vi "EELS Test V3.vi"() -> ()   [LabVIEW 2012]
uses:
  <instrlib>/Quantum Composers 9000 Series/Quantum Composers 9000 Series.lvlib
panel:
  in  "Continuous Wave":bool=TRUE
  out "Spectrum Measurement Recipe ID":dbl
  out "Dates":T1={"Measurement Date"=timestamp(3619697085.7529235 s since 1904-01-01), "Session Date"=timestamp(0 s since 1904-01-01)}
  in  "DeviceInfo":T2={"Cavity Length (um)"="1500", "Cavity Width (um)"="10", "X Position"="1", "Part Name"="0-0-1-10-1500"}
  out "Processing Recipe ID":dbl
  out "Spectrum Parameters":T3={"Peak Wavelengh (dbm)"="", "Peak Power (dbm)"="", "FWHM (nm)"="", "Input Current (mA)"="", "Measurement Recipe ID"=1.0, "Processing Recipe ID"=0.0, "Temperature"=0.0}
  out "LIV Array":dbl[][](array[numeric])=[[1.304, 1.304, 1.304, 1.304, 1.304, 1.304, 1.304, 1.303, 1.303, 1.302, 1.302, 1.302, 1.302, 1.302, 1.301, 1.301, 1.301, 1.301, 1.3, 1.3, 1.3, 1.3, 1.299, 1.299, 1.3, 1.299, 1.299, 1.298, 1.298, 1.298, 1.298, 1.296, 1.296, 1.296, 1.296, 1.296, 1.295, 1.295, 1.295, 1.295, 1.294, 1.294, 1.294, 1.294, 1.294, 1.292, 1.292, 1.292, 1.292, 1.29, 1.29, 1.29, 1.29, 1.29, 1.289, 1.289, 1.289, 1.289, 1.288, 1.287, 1.287, 1.287, 1.285, 1.285, 1.285, 1.285, 1.285, 1.283, 1.283, 1.283, 1.284, 1.282, 1.282, 1.282, 1.282, 1.282, 1.28, 1.28, 1.28, 1.28, 1.28, 1.278, 1.278, 1.278, 1.278, 1.276, 1.276, 1.276, 1.276, 1.274, 1.274, 1.274, 1.274, 1.274, 1.272, 1.272, 1.272, 1.272, 1.269, 1.269, 1.269, 1.269, 1.269, 1.267, 1.267, 1.267, 1.268, 1.265, 1.265, 1.265, 1.265, 1.265, 1.263, 1.263, 1.263, 1.263, 1.261, 1.261, 1.261, 1.261, 1.261, 1.259, 1.259, 1.259, 1.259, 1.256, 1.256, 1.256, 1.256, 1.256, 1.254, 1.254, 1.254, 1.254, 1.252, 1.252, 1.252, 1.252, 1.25, 1.249, 1.249, 1.249, 1.249, 1.248, 1.248, 1.248, 1.247, 1.245, 1.245, 1.245, 1.245, 1.245, 1.243, 1.243, 1.243, 1.243, 1.241, 1.241, 1.241, 1.241, 1.241, 1.238, 1.238, 1.238, 1.238, 1.236, 1.236, 1.236, 1.236, 1.236, 1.234, 1.234, 1.234, 1.234, 1.232, 1.232, 1.232, 1.232, 1.229, 1.229, 1.229, 1.229, 1.229, 1.227, 1.227, 1.227, 1.227, 1.227, 1.225, 1.225, 1.225, 1.225, 1.223, 1.223, 1.222, 1.223, 1.223, 1.22, 1.22, 1.22, 1.22], [216.66666666666669, 216.66666666666669, 216.66666666666669, 216.66666666666669, 216.66666666666669, 220.0, 220.0, 220.0, 220.0, 223.33333333333334, 226.66666666666666, 226.66666666666666, 223.33333333333334, 223.33333333333334, 230.00000000000003, 230.00000000000003, 230.00000000000003, 230.00000000000003, 233.33333333333334, 233.33333333333334, 233.33333333333334, 233.33333333333334, 236.66666666666666, 236.66666666666666, 236.66666666666666, 236.66666666666666, 236.66666666666666, 243.33333333333334, 243.33333333333334, 243.33333333333334, 243.33333333333334, 246.66666666666669, 246.66666666666669, 246.66666666666669, 246.66666666666669, 246.66666666666669, 250.0, 250.0, 250.0, 250.0, 256.6666666666667, 256.6666666666667, 256.6666666666667, 256.6666666666667, 256.6666666666667, 260.0, 260.0, 260.0, 260.0, 263.33333333333337, 263.33333333333337, 263.33333333333337, 263.33333333333337, 263.33333333333337, 270.0, 270.0, 270.0, 270.0, 273.3333333333333, 273.3333333333333, 273.3333333333333, 273.3333333333333, 276.6666666666667, 276.6666666666667, 276.6666666666667, 276.6666666666667, 276.6666666666667, 283.33333333333337, 283.33333333333337, 280.0, 283.33333333333337, 286.6666666666667, 286.6666666666667, 286.6666666666667, 286.6666666666667, 286.6666666666667, 290.0, 290.0, 290.0, 290.0, 290.0, 293.33333333333337, 293.33333333333337, 293.33333333333337, 293.33333333333337, 300.0, 300.0, 300.0, 300.0, 303.3333333333333, 303.3333333333333, 303.3333333333333, 303.3333333333333, 303.3333333333333, 306.66666666666663, 306.66666666666663, 306.66666666666663, 306.66666666666663, 313.33333333333337, 313.33333333333337, 313.33333333333337, 313.33333333333337, 313.33333333333337, 316.6666666666667, 316.6666666666667, 316.6666666666667, 316.6666666666667, 320.0, 320.0, 320.0, 320.0, 320.0, 326.6666666666667, 326.6666666666667, 326.6666666666667, 326.6666666666667, 330.0, 330.0, 330.0, 330.0, 330.0, 333.33333333333337, 333.33333333333337, 333.33333333333337, 333.33333333333337, 340.0, 340.0, 340.0, 340.0, 340.0, 343.33333333333337, 343.33333333333337, 343.33333333333337, 343.33333333333337, 346.6666666666667, 346.6666666666667, 346.6666666666667, 346.6666666666667, 353.3333333333333, 353.3333333333333, 353.3333333333333, 353.3333333333333, 353.3333333333333, 356.66666666666663, 356.66666666666663, 356.66666666666663, 356.66666666666663, 360.00000000000006, 360.00000000000006, 360.00000000000006, 360.00000000000006, 360.00000000000006, 363.33333333333337, 363.33333333333337, 363.33333333333337, 363.33333333333337, 370.0, 370.0, 370.0, 370.0, 370.0, 373.3333333333333, 373.3333333333333, 373.3333333333333, 373.3333333333333, 376.6666666666667, 376.6666666666667, 376.6666666666667, 376.6666666666667, 376.6666666666667, 383.33333333333337, 383.33333333333337, 383.33333333333337, 383.33333333333337, 386.6666666666667, 386.6666666666667, 386.6666666666667, 386.6666666666667, 390.0, 390.0, 390.0, 390.0, 390.0, 396.6666666666667, 396.6666666666667, 396.6666666666667, 396.6666666666667, 396.6666666666667, 400.0, 400.0, 400.0, 400.0, 406.6666666666667, 403.3333333333333, 403.3333333333333, 403.3333333333333, 403.3333333333333, 410.00000000000006, 410.00000000000006, 410.00000000000006, 410.00000000000006], [0.025723833333333338, 0.025771333333333334, 0.025723833333333338, 0.025700133333333337, 0.025723833333333338, 0.02764603333333333, 0.02766973333333333, 0.02764603333333333, 0.02766973333333333, 0.029568200000000003, 0.029568200000000003, 0.0295207, 0.029568200000000003, 0.0295919, 0.0316802, 0.0316802, 0.0316802, 0.03165646666666667, 0.03395833333333333, 0.03393466666666667, 0.03393466666666667, 0.033982000000000005, 0.036331333333333334, 0.036331333333333334, 0.036355000000000005, 0.036355000000000005, 0.03630766666666667, 0.038941666666666666, 0.039013, 0.038941666666666666, 0.03896533333333333, 0.041931666666666666, 0.041931666666666666, 0.041931666666666666, 0.041979333333333334, 0.042003, 0.04549133333333334, 0.04549133333333334, 0.04542, 0.04546766666666667, 0.050190000000000005, 0.050166333333333334, 0.050166333333333334, 0.050095, 0.05011866666666667, 0.05785466666666667, 0.057926, 0.05783100000000001, 0.05785466666666667, 0.094637, 0.09451833333333334, 0.09373533333333334, 0.09423366666666667, 0.094281, 0.259421, 0.26146166666666665, 0.26518733333333333, 0.2657333333333333, 0.5063133333333334, 0.5069066666666667, 0.51006, 0.50268, 0.7989800000000001, 0.7944466666666667, 0.7896766666666666, 0.7862133333333332, 0.78664, 1.13296, 1.1350733333333334, 1.1380633333333332, 1.1477933333333334, 1.4813300000000003, 1.48841, 1.4895933333333333, 1.4940766666666667, 1.48912, 1.9095566666666668, 1.90578, 1.8970466666666668, 1.89445, 1.8982266666666667, 2.34109, 2.3356600000000003, 2.3382566666666666, 2.3389666666666664, 2.81795, 2.83778, 2.8368333333333333, 2.8559566666666667, 3.3503000000000003, 3.344866666666667, 3.341066666666667, 3.3392, 3.335633333333333, 3.8592333333333335, 3.864666666666667, 3.8618333333333337, 3.8595, 4.399366666666667, 4.393933333333333, 4.3963, 4.397966666666667, 4.399133333333333, 4.958866666666666, 4.962166666666667, 4.9761, 4.977733333333334, 5.538166666666667, 5.536033333333334, 5.5365, 5.5436, 5.5311, 6.106366666666666, 6.103800000000001, 6.095766666666667, 6.0974, 6.676966666666666, 6.6828666666666665, 6.690433333333333, 6.687600000000001, 6.693966666666666, 7.294766666666667, 7.293333333333333, 7.291666666666667, 7.287433333333334, 7.871233333333334, 7.878066666666667, 7.8729000000000005, 7.8729000000000005, 7.864633333333334, 8.461866666666667, 8.467766666666668, 8.455266666666667, 8.465900000000001, 9.044733333333333, 9.0492, 9.0622, 9.052033333333336, 9.645299999999999, 9.661566666666666, 9.650966666666669, 9.659433333333334, 9.656866666666666, 10.165566666666667, 10.169366666666667, 10.176666666666668, 10.1781, 10.767566666666667, 10.786433333333335, 10.7666, 10.7678, 10.763766666666665, 11.351833333333333, 11.3431, 11.329166666666666, 11.334833333333334, 11.923100000000002, 11.913666666666668, 11.905166666666666, 11.904933333333334, 11.9002, 12.472433333333333, 12.484966666666669, 12.479066666666666, 12.474100000000002, 13.1072, 13.093033333333334, 13.1072, 13.121366666666669, 13.097766666666667, 13.723166666666668, 13.711366666666667, 13.6854, 13.718433333333333, 14.334400000000002, 14.315500000000002, 14.282466666666666, 14.308433333333333, 14.988100000000001, 14.929100000000002, 14.947966666666668, 14.962133333333334, 14.933800000000002, 15.799900000000001, 15.788133333333334, 15.804633333333333, 15.804633333333333, 15.764533333333334, 16.9209, 16.939766666666667, 16.9445, 16.913833333333333, 17.938033333333333, 17.869600000000002, 17.909733333333335, 17.8932, 17.900266666666663, 18.6838, 18.6413, 18.672, 18.620066666666666]]
  in  "Operator":string="sswifter"
  out "LIV Parameters":T4={"Threshold Current (mA)"=0.0, "Threshold Voltage (V)"=1.288, "Slope Efficiency"=1.0882708585247884, "Temperature"=15.0, "Measurement Recipe ID"=1.0, "Processing Recipe ID"=0.0}
  in  "update wafer info":bool
  in  "WaferInfo":T5={"WaferName"="TGR-163-1", "Scribe"="J3393-115", "Structure"="1068.1.1", "Lot"="SJC_ENG_375_4-GaAs", "Mask"="PH002"}
  in  "vi find peak":path=path "C:/Users/test_QE/Desktop/NanoMAX SubVI/NanoMAX 1D Find Peak Power 3D.vi"
  in  "vi path piezosfine":path=path "C:/Users/test_QE/Desktop/NanoMAX SubVI/NanoMAX300 Align Fiber Piezos.vi"
  in  "vi path stepper fine":path=path "C:/Users/test_QE/Desktop/NanoMAX SubVI/NanoMAX300 Align Fiber Steppers.vi"
  out "intensity array":dbl[](array[numeric])
  out "Wavelength Array":dbl[](array[numeric])
  out "data step":dbl
  out "Current lambda":dbl
  out "Numeric":i32
  out "Piezo Refs":refnum<k7>[](array[refnum])
  out "Stepper Refs":refnum<k7>[](array[refnum])
  in  "stop":bool
  out "P array":dbl[](array[numeric])=[0.025723833333333338, 0.025771333333333334, 0.025723833333333338, 0.025700133333333337, 0.025723833333333338, 0.02764603333333333, 0.02766973333333333, 0.02764603333333333, 0.02766973333333333, 0.029568200000000003, 0.029568200000000003, 0.0295207, 0.029568200000000003, 0.0295919, 0.0316802, 0.0316802, 0.0316802, 0.03165646666666667, 0.03395833333333333, 0.03393466666666667, 0.03393466666666667, 0.033982000000000005, 0.036331333333333334, 0.036331333333333334, 0.036355000000000005, 0.036355000000000005, 0.03630766666666667, 0.038941666666666666, 0.039013, 0.038941666666666666, 0.03896533333333333, 0.041931666666666666, 0.041931666666666666, 0.041931666666666666, 0.041979333333333334, 0.042003, 0.04549133333333334, 0.04549133333333334, 0.04542, 0.04546766666666667, 0.050190000000000005, 0.050166333333333334, 0.050166333333333334, 0.050095, 0.05011866666666667, 0.05785466666666667, 0.057926, 0.05783100000000001, 0.05785466666666667, 0.094637, 0.09451833333333334, 0.09373533333333334, 0.09423366666666667, 0.094281, 0.259421, 0.26146166666666665, 0.26518733333333333, 0.2657333333333333, 0.5063133333333334, 0.5069066666666667, 0.51006, 0.50268, 0.7989800000000001, 0.7944466666666667, 0.7896766666666666, 0.7862133333333332, 0.78664, 1.13296, 1.1350733333333334, 1.1380633333333332, 1.1477933333333334, 1.4813300000000003, 1.48841, 1.4895933333333333, 1.4940766666666667, 1.48912, 1.9095566666666668, 1.90578, 1.8970466666666668, 1.89445, 1.8982266666666667, 2.34109, 2.3356600000000003, 2.3382566666666666, 2.3389666666666664, 2.81795, 2.83778, 2.8368333333333333, 2.8559566666666667, 3.3503000000000003, 3.344866666666667, 3.341066666666667, 3.3392, 3.335633333333333, 3.8592333333333335, 3.864666666666667, 3.8618333333333337, 3.8595, 4.399366666666667, 4.393933333333333, 4.3963, 4.397966666666667, 4.399133333333333, 4.958866666666666, 4.962166666666667, 4.9761, 4.977733333333334, 5.538166666666667, 5.536033333333334, 5.5365, 5.5436, 5.5311, 6.106366666666666, 6.103800000000001, 6.095766666666667, 6.0974, 6.676966666666666, 6.6828666666666665, 6.690433333333333, 6.687600000000001, 6.693966666666666, 7.294766666666667, 7.293333333333333, 7.291666666666667, 7.287433333333334, 7.871233333333334, 7.878066666666667, 7.8729000000000005, 7.8729000000000005, 7.864633333333334, 8.461866666666667, 8.467766666666668, 8.455266666666667, 8.465900000000001, 9.044733333333333, 9.0492, 9.0622, 9.052033333333336, 9.645299999999999, 9.661566666666666, 9.650966666666669, 9.659433333333334, 9.656866666666666, 10.165566666666667, 10.169366666666667, 10.176666666666668, 10.1781, 10.767566666666667, 10.786433333333335, 10.7666, 10.7678, 10.763766666666665, 11.351833333333333, 11.3431, 11.329166666666666, 11.334833333333334, 11.923100000000002, 11.913666666666668, 11.905166666666666, 11.904933333333334, 11.9002, 12.472433333333333, 12.484966666666669, 12.479066666666666, 12.474100000000002, 13.1072, 13.093033333333334, 13.1072, 13.121366666666669, 13.097766666666667, 13.723166666666668, 13.711366666666667, 13.6854, 13.718433333333333, 14.334400000000002, 14.315500000000002, 14.282466666666666, 14.308433333333333, 14.988100000000001, 14.929100000000002, 14.947966666666668, 14.962133333333334, 14.933800000000002, 15.799900000000001, 15.788133333333334, 15.804633333333333, 15.804633333333333, 15.764533333333334, 16.9209, 16.939766666666667, 16.9445, 16.913833333333333, 17.938033333333333, 17.869600000000002, 17.909733333333335, 17.8932, 17.900266666666663, 18.6838, 18.6413, 18.672, 18.620066666666666]
  out "I Array":dbl[](array[numeric])=[216.66666666666669, 216.66666666666669, 216.66666666666669, 216.66666666666669, 216.66666666666669, 220.0, 220.0, 220.0, 220.0, 223.33333333333334, 226.66666666666666, 226.66666666666666, 223.33333333333334, 223.33333333333334, 230.00000000000003, 230.00000000000003, 230.00000000000003, 230.00000000000003, 233.33333333333334, 233.33333333333334, 233.33333333333334, 233.33333333333334, 236.66666666666666, 236.66666666666666, 236.66666666666666, 236.66666666666666, 236.66666666666666, 243.33333333333334, 243.33333333333334, 243.33333333333334, 243.33333333333334, 246.66666666666669, 246.66666666666669, 246.66666666666669, 246.66666666666669, 246.66666666666669, 250.0, 250.0, 250.0, 250.0, 256.6666666666667, 256.6666666666667, 256.6666666666667, 256.6666666666667, 256.6666666666667, 260.0, 260.0, 260.0, 260.0, 263.33333333333337, 263.33333333333337, 263.33333333333337, 263.33333333333337, 263.33333333333337, 270.0, 270.0, 270.0, 270.0, 273.3333333333333, 273.3333333333333, 273.3333333333333, 273.3333333333333, 276.6666666666667, 276.6666666666667, 276.6666666666667, 276.6666666666667, 276.6666666666667, 283.33333333333337, 283.33333333333337, 280.0, 283.33333333333337, 286.6666666666667, 286.6666666666667, 286.6666666666667, 286.6666666666667, 286.6666666666667, 290.0, 290.0, 290.0, 290.0, 290.0, 293.33333333333337, 293.33333333333337, 293.33333333333337, 293.33333333333337, 300.0, 300.0, 300.0, 300.0, 303.3333333333333, 303.3333333333333, 303.3333333333333, 303.3333333333333, 303.3333333333333, 306.66666666666663, 306.66666666666663, 306.66666666666663, 306.66666666666663, 313.33333333333337, 313.33333333333337, 313.33333333333337, 313.33333333333337, 313.33333333333337, 316.6666666666667, 316.6666666666667, 316.6666666666667, 316.6666666666667, 320.0, 320.0, 320.0, 320.0, 320.0, 326.6666666666667, 326.6666666666667, 326.6666666666667, 326.6666666666667, 330.0, 330.0, 330.0, 330.0, 330.0, 333.33333333333337, 333.33333333333337, 333.33333333333337, 333.33333333333337, 340.0, 340.0, 340.0, 340.0, 340.0, 343.33333333333337, 343.33333333333337, 343.33333333333337, 343.33333333333337, 346.6666666666667, 346.6666666666667, 346.6666666666667, 346.6666666666667, 353.3333333333333, 353.3333333333333, 353.3333333333333, 353.3333333333333, 353.3333333333333, 356.66666666666663, 356.66666666666663, 356.66666666666663, 356.66666666666663, 360.00000000000006, 360.00000000000006, 360.00000000000006, 360.00000000000006, 360.00000000000006, 363.33333333333337, 363.33333333333337, 363.33333333333337, 363.33333333333337, 370.0, 370.0, 370.0, 370.0, 370.0, 373.3333333333333, 373.3333333333333, 373.3333333333333, 373.3333333333333, 376.6666666666667, 376.6666666666667, 376.6666666666667, 376.6666666666667, 376.6666666666667, 383.33333333333337, 383.33333333333337, 383.33333333333337, 383.33333333333337, 386.6666666666667, 386.6666666666667, 386.6666666666667, 386.6666666666667, 390.0, 390.0, 390.0, 390.0, 390.0, 396.6666666666667, 396.6666666666667, 396.6666666666667, 396.6666666666667, 396.6666666666667, 400.0, 400.0, 400.0, 400.0, 406.6666666666667, 403.3333333333333, 403.3333333333333, 403.3333333333333, 403.3333333333333, 410.00000000000006, 410.00000000000006, 410.00000000000006, 410.00000000000006]
  out "V Array":dbl[](array[numeric])=[1.304, 1.304, 1.304, 1.304, 1.304, 1.304, 1.304, 1.303, 1.303, 1.302, 1.302, 1.302, 1.302, 1.302, 1.301, 1.301, 1.301, 1.301, 1.3, 1.3, 1.3, 1.3, 1.299, 1.299, 1.3, 1.299, 1.299, 1.298, 1.298, 1.298, 1.298, 1.296, 1.296, 1.296, 1.296, 1.296, 1.295, 1.295, 1.295, 1.295, 1.294, 1.294, 1.294, 1.294, 1.294, 1.292, 1.292, 1.292, 1.292, 1.29, 1.29, 1.29, 1.29, 1.29, 1.289, 1.289, 1.289, 1.289, 1.288, 1.287, 1.287, 1.287, 1.285, 1.285, 1.285, 1.285, 1.285, 1.283, 1.283, 1.283, 1.284, 1.282, 1.282, 1.282, 1.282, 1.282, 1.28, 1.28, 1.28, 1.28, 1.28, 1.278, 1.278, 1.278, 1.278, 1.276, 1.276, 1.276, 1.276, 1.274, 1.274, 1.274, 1.274, 1.274, 1.272, 1.272, 1.272, 1.272, 1.269, 1.269, 1.269, 1.269, 1.269, 1.267, 1.267, 1.267, 1.268, 1.265, 1.265, 1.265, 1.265, 1.265, 1.263, 1.263, 1.263, 1.263, 1.261, 1.261, 1.261, 1.261, 1.261, 1.259, 1.259, 1.259, 1.259, 1.256, 1.256, 1.256, 1.256, 1.256, 1.254, 1.254, 1.254, 1.254, 1.252, 1.252, 1.252, 1.252, 1.25, 1.249, 1.249, 1.249, 1.249, 1.248, 1.248, 1.248, 1.247, 1.245, 1.245, 1.245, 1.245, 1.245, 1.243, 1.243, 1.243, 1.243, 1.241, 1.241, 1.241, 1.241, 1.241, 1.238, 1.238, 1.238, 1.238, 1.236, 1.236, 1.236, 1.236, 1.236, 1.234, 1.234, 1.234, 1.234, 1.232, 1.232, 1.232, 1.232, 1.229, 1.229, 1.229, 1.229, 1.229, 1.227, 1.227, 1.227, 1.227, 1.227, 1.225, 1.225, 1.225, 1.225, 1.223, 1.223, 1.222, 1.223, 1.223, 1.22, 1.22, 1.22, 1.22]
  in  "?":T6(tab)=enum."Power"
  in  "Comments on Spectrum":string="testing"
  in  "Step Size (nm)":string="1"
  out "FWHM (nm)":string
  in  "Save Spectrum to File":bool
  out "Spectrum Readout":cluster{dbl[], "array type (2D Dbl)":dbl[]}(graph)
  in  "Preform Sweep":bool
  in  "Update OSA Settings":bool
  in  "Start Wavelength (nm)":string="1250"
  in  "Stop Wavelength (nm)":string="1400"
  in  "Sensitivity (dBm)":string="-40"
  in  "Resolution Bandwidth (nm)":string="1"
  out "OSA Error":errorcluster
  out "Peak Wavelength (nm)":string
  out "Peak Intensity (dBm)":string
  in  "byte count":u32=50000
  in  "Spectrum File Location":path=path "C:/Users/test_QE/Desktop/EELS Data/Spectrum Data"
  out "Spectrum Recipe Description":string
  in  "spectrum measuement presets 2":bool
  out "Current Processing Recipe":T7={"Soldering Material"="InSn", "Soldering Method"="Hand Soldered", "Company"="SJC", "Submount Type"="Flat Bar", "Submount Material"="Copper", "Comments"="soldered by eye on chuck", "Recipe ID"="1"}
  in  "select processing recipe":bool
  out "Measured Average Current":dbl
  out "Calculated Peak Current":dbl
  in  "Current Step Delay":dbl=1.0
  out "Duty Cycle (Update in Settings)":dbl=0.03
  in  "LIV Measurement Comments":string
  in  "measuement presets":bool
  out "Current Setpoint":dbl=100.0
  in  "start sweep":bool
  in  "Wavelength":dbl=1350.0
  in  "Step Size":dbl=1.0
  in  "End Current":dbl=300.0
  in  "Start Current":dbl=100.0
  out "# Data Points":dbl=201.0
  out "Current Vs. Power":cluster{"Y":dbl[], "Y":dbl[]}[](graph) caption="XY Graph"
  out "Voltage Vs. Current":cluster{"Y":dbl[], "Y":dbl[]}[](graph)=[{"Y"=[1.304, 1.304, 1.304, 1.304, 1.304, 1.304, 1.304, 1.303, 1.303, 1.302, 1.302, 1.302, 1.302, 1.302, 1.301, 1.301, 1.301, 1.301, 1.3, 1.3, 1.3, 1.3, 1.299, 1.299, 1.3, 1.299, 1.299, 1.298, 1.298, 1.298, 1.298, 1.296, 1.296, 1.296, 1.296, 1.296, 1.295, 1.295, 1.295, 1.295, 1.294, 1.294, 1.294, 1.294, 1.294, 1.292, 1.292, 1.292, 1.292, 1.29, 1.29, 1.29, 1.29, 1.29, 1.289, 1.289, 1.289, 1.289, 1.288, 1.287, 1.287, 1.287, 1.285, 1.285, 1.285, 1.285, 1.285, 1.283, 1.283, 1.283, 1.284, 1.282, 1.282, 1.282, 1.282, 1.282, 1.28, 1.28, 1.28, 1.28, 1.28, 1.278, 1.278, 1.278, 1.278, 1.276, 1.276, 1.276, 1.276, 1.274, 1.274, 1.274, 1.274, 1.274, 1.272, 1.272, 1.272, 1.272, 1.269, 1.269, 1.269, 1.269, 1.269, 1.267, 1.267, 1.267, 1.268, 1.265, 1.265, 1.265, 1.265, 1.265, 1.263, 1.263, 1.263, 1.263, 1.261, 1.261, 1.261, 1.261, 1.261, 1.259, 1.259, 1.259, 1.259, 1.256, 1.256, 1.256, 1.256, 1.256, 1.254, 1.254, 1.254, 1.254, 1.252, 1.252, 1.252, 1.252, 1.25, 1.249, 1.249, 1.249, 1.249, 1.248, 1.248, 1.248, 1.247, 1.245, 1.245, 1.245, 1.245, 1.245, 1.243, 1.243, 1.243, 1.243, 1.241, 1.241, 1.241, 1.241, 1.241, 1.238, 1.238, 1.238, 1.238, 1.236, 1.236, 1.236, 1.236, 1.236, 1.234, 1.234, 1.234, 1.234, 1.232, 1.232, 1.232, 1.232, 1.229, 1.229, 1.229, 1.229, 1.229, 1.227, 1.227, 1.227, 1.227, 1.227, 1.225, 1.225, 1.225, 1.225, 1.223, 1.223, 1.222, 1.223, 1.223, 1.22, 1.22, 1.22, 1.22], "Y"=[216.66666666666669, 216.66666666666669, 216.66666666666669, 216.66666666666669, 216.66666666666669, 220.0, 220.0, 220.0, 220.0, 223.33333333333334, 226.66666666666666, 226.66666666666666, 223.33333333333334, 223.33333333333334, 230.00000000000003, 230.00000000000003, 230.00000000000003, 230.00000000000003, 233.33333333333334, 233.33333333333334, 233.33333333333334, 233.33333333333334, 236.66666666666666, 236.66666666666666, 236.66666666666666, 236.66666666666666, 236.66666666666666, 243.33333333333334, 243.33333333333334, 243.33333333333334, 243.33333333333334, 246.66666666666669, 246.66666666666669, 246.66666666666669, 246.66666666666669, 246.66666666666669, 250.0, 250.0, 250.0, 250.0, 256.6666666666667, 256.6666666666667, 256.6666666666667, 256.6666666666667, 256.6666666666667, 260.0, 260.0, 260.0, 260.0, 263.33333333333337, 263.33333333333337, 263.33333333333337, 263.33333333333337, 263.33333333333337, 270.0, 270.0, 270.0, 270.0, 273.3333333333333, 273.3333333333333, 273.3333333333333, 273.3333333333333, 276.6666666666667, 276.6666666666667, 276.6666666666667, 276.6666666666667, 276.6666666666667, 283.33333333333337, 283.33333333333337, 280.0, 283.33333333333337, 286.6666666666667, 286.6666666666667, 286.6666666666667, 286.6666666666667, 286.6666666666667, 290.0, 290.0, 290.0, 290.0, 290.0, 293.33333333333337, 293.33333333333337, 293.33333333333337, 293.33333333333337, 300.0, 300.0, 300.0, 300.0, 303.3333333333333, 303.3333333333333, 303.3333333333333, 303.3333333333333, 303.3333333333333, 306.66666666666663, 306.66666666666663, 306.66666666666663, 306.66666666666663, 313.33333333333337, 313.33333333333337, 313.33333333333337, 313.33333333333337, 313.33333333333337, 316.6666666666667, 316.6666666666667, 316.6666666666667, 316.6666666666667, 320.0, 320.0, 320.0, 320.0, 320.0, 326.6666666666667, 326.6666666666667, 326.6666666666667, 326.6666666666667, 330.0, 330.0, 330.0, 330.0, 330.0, 333.33333333333337, 333.33333333333337, 333.33333333333337, 333.33333333333337, 340.0, 340.0, 340.0, 340.0, 340.0, 343.33333333333337, 343.33333333333337, 343.33333333333337, 343.33333333333337, 346.6666666666667, 346.6666666666667, 346.6666666666667, 346.6666666666667, 353.3333333333333, 353.3333333333333, 353.3333333333333, 353.3333333333333, 353.3333333333333, 356.66666666666663, 356.66666666666663, 356.66666666666663, 356.66666666666663, 360.00000000000006, 360.00000000000006, 360.00000000000006, 360.00000000000006, 360.00000000000006, 363.33333333333337, 363.33333333333337, 363.33333333333337, 363.33333333333337, 370.0, 370.0, 370.0, 370.0, 370.0, 373.3333333333333, 373.3333333333333, 373.3333333333333, 373.3333333333333, 376.6666666666667, 376.6666666666667, 376.6666666666667, 376.6666666666667, 376.6666666666667, 383.33333333333337, 383.33333333333337, 383.33333333333337, 383.33333333333337, 386.6666666666667, 386.6666666666667, 386.6666666666667, 386.6666666666667, 390.0, 390.0, 390.0, 390.0, 390.0, 396.6666666666667, 396.6666666666667, 396.6666666666667, 396.6666666666667, 396.6666666666667, 400.0, 400.0, 400.0, 400.0, 406.6666666666667, 403.3333333333333, 403.3333333333333, 403.3333333333333, 403.3333333333333, 410.00000000000006, 410.00000000000006, 410.00000000000006, 410.00000000000006]}] caption="XY Graph"
  out "DQE":dbl=1.0882708585247884
  out "Threshold Current (mA)":dbl
  in  "Counts per Data Point":i32=10
  in  "Time per Count (s)":dbl=0.001
  out "Estimated Sweep Time":dbl=203.01
  out "Threshold Voltage (V)":dbl=1.288
  out "Max Power (mW)":dbl=18.6838
  out "Current @ Max Power":dbl=410.00000000000006
  out "energy/photon (eV)":dbl=0.9188888888888889
  out "slope efficincy":dbl=1.0
  out "Least Squares Residue":dbl
  in  "Sweep save path":path=path "C:/Users/test_QE/Desktop/EELS Data/LIV Data"
  out "Recipe Description":string="100-350 CW 5ma step"
  in  "begin temp series":bool
  in  "remove temp list":bool
  in  "clear list":bool
  in  "TEMP DESIRED":string
  in  "TEMP LIST":i32(listbox)
  in  "add temp to list":bool
  out "Current v. Power":cluster{dbl[], dbl[]}[](graph)
  out "Voltage v. Current":cluster{"x":dbl[], "y3":dbl[]}[](graph)
  in  "Tab Control 2":T8(tab)
  out "Y Axis Profile":T9(graph)
  out "Position of Max Power Y":sgl
  out "Max Power Y":dbl
  out "Z Axis Profile":T9(graph)
  out "Max Power Z":dbl
  out "Position of Max Power Z":sgl
  out "X Axis Profile":T9(graph)
  out "Position of Max Power X":sgl
  out "Max Power X":dbl
  in  "X Distance for YZ Scan(mm)":sgl=3.75
  in  "Move to Loading Position":bool
  in  "Home Stepper Motors":bool
  in  "auto align":bool
  in  "Find Peak":bool
  in  "auto align step fine":bool
  in  "auto align piezo fine":bool
  in  "MG17Piezo Z Axis":refnum<k7>(container)
  in  "MG17Piezo Y Axis":refnum<k7>(container)
  in  "MG17Piezo X Axis":refnum<k7>(container)
  in  "Enable Manual Stage Control":bool
  in  "Stepper Z Axis":refnum<k7>(container)
  in  "Stepper X Axis":refnum<k7>(container)
  in  "Stepper Y Axis":refnum<k7>(container)
  in  "Exit Manual Stage Control":bool
  in  "Serial Numbers Piezo":T10={"MotorA HWSerialNum"=91877934, "Motor B HWSerialNum"=91877935, "Motor C HWSerialNum"=91877936}
  in  "Serial Numbers Stepper Motors":T10={"MotorA HWSerialNum"=90877891, "Motor B HWSerialNum"=90877892, "Motor C HWSerialNum"=90877893}
  in  "Temptronics update":bool
  in  "Delay Width (ms)":dbl=0.095
  in  "Pulse Width (ms)":dbl=0.005
  out "Duty Cycle":dbl=1.0
  in  "pulse generator update":bool
  in  "Laser Output":bool
  in  "power meter":bool
  in  "?":bool
  in  "Beep?":bool
  in  "COM Port":i16=3
  out "Arroyo VISA":refnum<visa-resource-name>="ASRL3::INSTR"
  in  "Laser Current Setpoint":dbl
  in  "Thorlabs PM100 VISA":refnum<visa-resource-name>="USB0::0x1313::0x8075::P5000840::INSTR" caption="resource name"
  out "Power":dbl
  out "Current":dbl
  in  "Quantum Composers VISA":refnum<visa-resource-name>="GPIB0::5::INSTR"
  in  "State (T:Enabled)":bool=TRUE
  in  "Channel (1:Chan A)":i32(ring)=1 items=["System (To)", "Channel A", "Channel B", "Channel C", "Channel D", "Channel E", "Channel F", "Channel G", "Channel H"]
  in  "TEC Output":bool
  in  "COM Port VISA":refnum<visa-resource-name>="COM3"
  in  "TEC Temperature Setpoint":dbl=25.0
  in  "Wavelength (0.0)":dbl=1350.0
  out "Instrument Errors":errorcluster
  in  "Level":T11(ring)=enum."Adjustable"
  in  "Adjustable":dbl=5.0 format="%.3p"
  in  "Temptronic VISA":refnum<visa-resource-name>="GPIB0::9::INSTR"
  in  "Temp Setpoint":string="15"
  out "Current Temp":string="24"
  in  "Power Unit (Watt)":i16(ring) items=["Watt", "dBm"]
  in  "Power Autorange Mode":u16(ring)=1 caption="Power Autorange Mode (ON)" items=["ON"=1, "OFF"=0]
  in  "Agilent OSA Visa":refnum<visa-resource-name>="GPIB0::23::INSTR"
  out "Agilent IDN Query":string="AGILE"
  out "Status":string="idle"
  out "error out":errorcluster
  # "EELS TESTING"
  # "Dont change this stuff"
  # "OSA Sweep"
  # "Current Sweep"
  # "Sweep Settings"
  # "Calculations"
  # "Current v. Power"
  # "Temperature Series"
  # "Voltage v. Current"
  # "(Sweep Settings Same as in Power Tab)"
  # "This is for Aligning The Integrating Sphere"
  # "Directions\n\n1) Move Chuck away from stage\n\n2) Home stepper motors and load integrating sphere\n\n3) Move to Loading Position (X-4, Y=Z=2). This allows for maximal \nalignment motion while ensuring the sphere doesn't scrape the chuck\n\n4) Move chuck with laser bar forward until almost touching the opening to the\nsphere, and set needle probes\n\n4) Set X distance for YZ scan (Usually 3<x<4)\n\n5) Press Auto Align"
  # "This is for aligning the GRIN Collimator. It has a resolution of ~1um"
  # "Directions\n\n1) Move Chuck away from stage\n\n2) Home stepper motors and load GRIN Collimator\n\n3) Move to Loading Position (X-4, Y=Z=2). This allows for maximal alignment motion while ensuring the GRIN doesn't scrape the chuck\n\n4) Move chuck with laser bar forward until almost touching the opening to the sphere, and set needle probes\n\n5) Turn on laser and align by eye using Manual Stage Controls tab and the Newport manual stage - maximize signal by eye\n\n6) Run FIND PEAK\n\n\n\n\n\nNOTE: This will occasionally pop up an error. I cannot figure out how to fix this, but if you dismiss the error the program will still run fine."
  # "Thorlabs Power Meter"
  # "Pulse Generator"
  # "Temptronic Chuck Control"
  # "Laser Driver"
  # "Note: Ignore PM100D Initialize Error"
  # "Agilent OSA"
  # "Standard Operating Procedures"
  # "LIV Measurement\n\n1) Mount Laser bar and align integrating sphere (see stage alignment)\n\n2) Select Meaurement Preset. If there is a preset that matches the measurement you wish to take, select that. If not, select the closest one and modify the parameters to fit your needs\n\n3) Enter comments that describe the experiment and any unusual parameters or circumstances present\n\n4) Ensure that the WaferInfo and DeviceInfor (left) are correct.\n\n5) Select \"Start Sweep\" and wait for the operation to complete\n\n6) If you changed the parameters, it will ask you to describe a new recipe. Enter comments that describe the recipe and hit OK\n\n7) The sweep is complete, the data is automatically saved to C:\\Users\\test_QE\\Desktop\\EELS Data\\LIV Data"
  # "Spectrum Measurement\n\n1) Mount Laser bar and align GRIN collimator (see stage alignment)\n\n2) Select Meaurement Preset. If there is a preset that matches the measurement you wish to take, select that. If not, select the closest one and modify the parameters to fit your needs. Then hit \"Update OSA settings\" to apply these changes.\n\nNOTE: If you type in changes but do not hit the update OSA button, the changes will not be applied and the sweep won't do what you think it does.\n\n3) Enter comments that describe the experiment and any unusual parameters or circumstances present\n\n4) Ensure that the WaferInfo and DeviceInfor (left) are correct.\n\n5) Select \"Preform Sweep\" and wait for the operation to complete. The sweep will be displayed on the graph. If you would like to save the sweep - click Save Spectrum to File\n\n6) If you changed the parameters, it will ask you to describe a new recipe. Enter comments that describe the recipe and hit OK\n\n7) The sweep is complete, the data is automatically saved to C:\\Users\\test_QE\\Desktop\\EELS Data\\Spectrum Data"
  # "Temperature Series\n\n1) Mount Laser bar and align Integrating Sphere (see stage alignment)\n\n2)Repeat steps 2-4 from LIV Measurement in Power tab. This will set the settings for each individual sweep\n\n3) Populate the temperature list with the temperatures you would like to be measured. Suggested temperatures are between 15C and 85 C. It is preferable to put the temperatures in ascending order\n\n4) Click begin series. The sweeps will run back to back.\n\n6) If you changed the parameters, it will ask you to describe a new recipe after the first sweep. Enter comments that describe the recipe and hit OK\n\n7) Once the sweep is complete, the data is automatically saved to C:\\Users\\test_QE\\Desktop\\EELS Data\\LIV Data. Each sweep will be saved to its own IV file"
  # "Upload Data to Local DB\n\n1) Move desired data to C:\\Users\\test_QE\\Desktop\\Local Database\\UPLOADS. Duplicates are OK, they will just be ignored\n\n2) Open Anaconda Command Prompt. This can be done by clicking the windows button in the bottom left and typing \"Anaconda\" into the search bar, and selecting Anaconda Command Prompt\n\n3)  Type in \"cd Desktop/Local Python Code\" and hit enter (not including quotation marks)\n\n4) Type in \"python UploadToLocalDB.py\" and hit enter\n\n5) Messages should appear in the console indicating the success or failure of the upload"
  # "1) Everything is frozen, the buttons are not responding even though the program is running.\n\n-> Make sure the \"Manual Stage Controls\" are off. Unfortunately, while those are running, the rest of the program holds until they are shut off.\n\n-> Labview could be in a recursion loop or waiting for an instrument response. If problems persist, force quit labview and restart the program"
  # "6) TEC won't turn on at all\n\n->There is a power switch in the back that also needs to be flipped in order for the TEC to turn on"
  # "7)  Stage is not moving properly - it says its at zero  and it clearly isn't (or similar issue)\n\n-> Try re-homing the stepper motors. This can be done under the stage alignment tab or manual stage control tab. Make sure the chuck is moved out of the way while you do this."
  # "2) I ran an IV sweep, and everything below 100mA doesn't look right.\n\n-> If you are using pulsed mode (not CW), the system can only operate at 100 mA or higher. This is because the minimal adjustable voltage for the quantum composers is 2V, which corresponds to a peak current of 100mA"
  # "8)  I input a certain range of currents, but the measured output was slightly different from these\n\n->In pulsed mode, the current is converted to a voltage for the quantum composers then reconverted to a current - so the conversion can slightly adjust the current level. Rest assured, however, that the measured current is actually correct even if it is different from the initial input"
  # "3) OSA is unresponsive and nothing is showing up on the screen\n\n-> This one is a bitch - check the problem by opening NI MAX (from windows menu), selecting the Agilent OSA (Devices and Interfaces, GPIB-USB-HS, scan for instruments, GPIB 23), and clicking \"Communicate with Instrument\" at the top of the screen. Then enter \"sys:err?\" into the text input and hit query. If the error mentions \"slit positioning system\" continue with the next step. Otherwise check the manual\n\n->If the error is the slit positining system, you need to factory preset and restart. Factory reset by typing in cal:alig:pres to the VISA communication window, then cycle power with the button on the front of the console. There is no guarantee that this will work, I had to do it 8 times or so to fix it last time."
  # "9) The threshold current is not even close to what it seems like it should be\n\n->If the power rolls over at high currents, the threshold current can be more difficult to calculate. The accuracy of the threshold current calculation can be ascertained by the R^2 value that describes the linear fit of the LI data."
  # "4) Laser is never really going above 100uW, or goes up and quickly drops back down, even though it is clearly conected\n\n-> The issue is most likely poor thermal contact. The laser bar could be soldered improperly, of there could be not enough arctic silver between the chuck and the submount. Try reapplying arctic silver\n\n->Some of the laser bars are just bad. Consider trying pulsed mode and see if you get a better result"
  # "5)Every time I try to turn the laser on, the laser driver clicks and an error message pops up saying \"V limit reached\"\n\n->This means the needle probes are an open circuit.  Check that they havent slipped and that the Anode probes are making good contact with the top of the bar and the Cathode is making contact with the submount.\n\n->It is possible that the breakout box is loose. After TURNING THE LASER OFF, check the connections of the breakout box with a voltmeter to ensure a good connection."
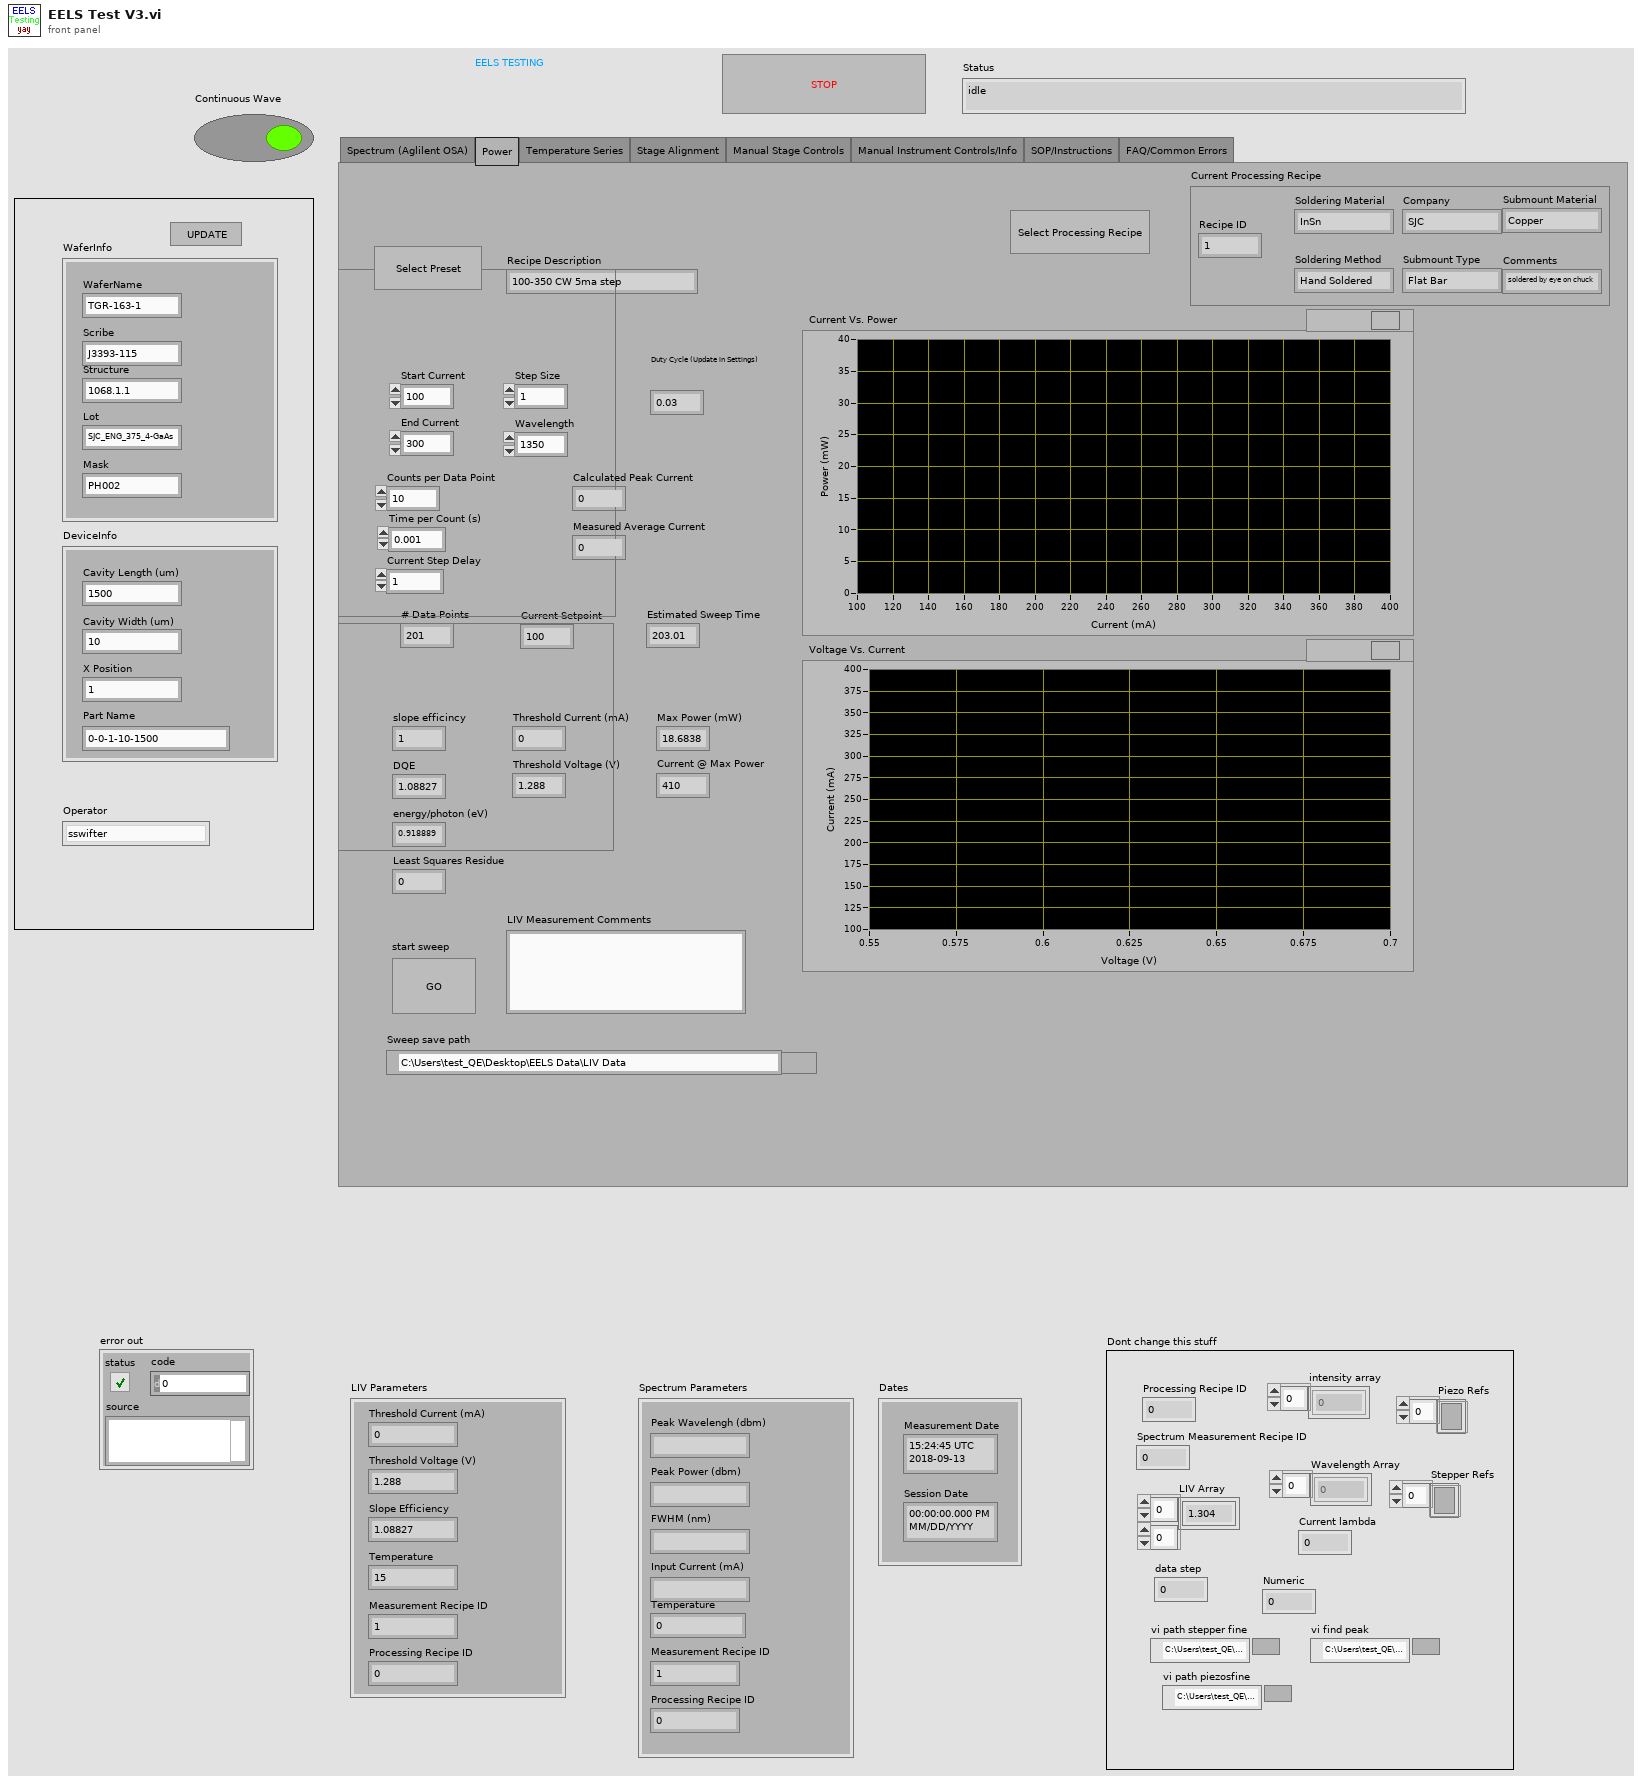
[diagram p1: front panel]
types:
  T1 = cluster{"Measurement Date":timestamp, "Session Date":timestamp}
  T2 = cluster{"Cavity Length (um)":string, "Cavity Width (um)":string, "X Position":string, "Part Name":string}
  T3 = cluster{"Peak Wavelengh (dbm)":string, "Peak Power (dbm)":string, "FWHM (nm)":string, "Input Current (mA)":string, "Measurement Recipe ID":dbl, "Processing Recipe ID":dbl, "Temperature":dbl}
  T4 = cluster{"Threshold Current (mA)":dbl, "Threshold Voltage (V)":dbl, "Slope Efficiency":dbl, "Temperature":dbl, "Measurement Recipe ID":dbl, "Processing Recipe ID":dbl}
  T5 = cluster{"WaferName":string, "Scribe":string, "Structure":string, "Lot":string, "Mask":string}
  T6 = enum32{"Spectrum (Aglilent OSA)", "Power", "Temperature Series", "Stage Alignment", "Manual Stage Controls", "Manual Instrument Controls/Info", "SOP/Instructions", "FAQ/Common Errors"}
  T7 = cluster{"Soldering Material":string, "Soldering Method":string, "Company":string, "Submount Type":string, "Submount Material":string, "Comments":string, "Recipe ID":string}
  T8 = enum32{"Coarse Alignment", "Peak Find VI", "Fine Alignment (Steppers)", "Fine Alignment (Piezos)"}
  T9 = cluster{"Position Array":sgl[], "Power Array":dbl[]}
  T10 = cluster{"MotorA HWSerialNum":i32, "Motor B HWSerialNum":i32, "Motor C HWSerialNum":i32}
  T11 = enum16{"TTL", "Adjustable", "35 Volt", "Optical"}
  T12 = cluster{"Start Current":string, "End Current":string, "Step Size":string, "# Data Points":string, "Points Averaged pr measurement":string, "Time Per Measurement":string, "Duty Cycle":string, "Pulse Width us":string, "Comments":string}
  T13 = cluster{"Recipe ID":string, "Start Wavelength":string, "End Wavelength":string, "Step Size":string, "Resolution Bandwidth":string, "Sensitivity":string, "Comments":string}
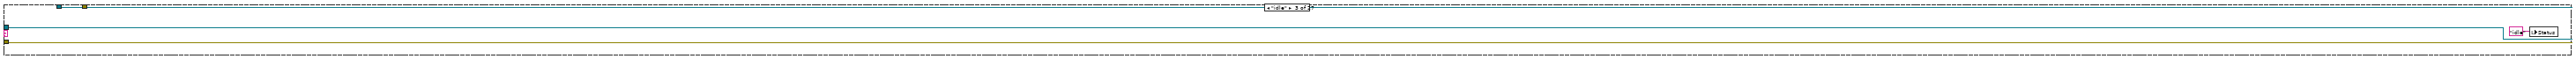
[diagram p4: hidden frame]
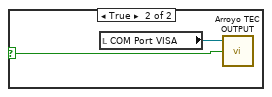
[diagram p6: hidden frame]
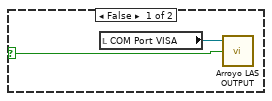
[diagram p7: hidden frame]
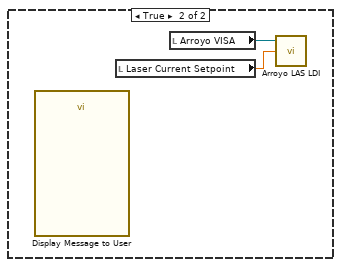
[diagram p8: hidden frame]
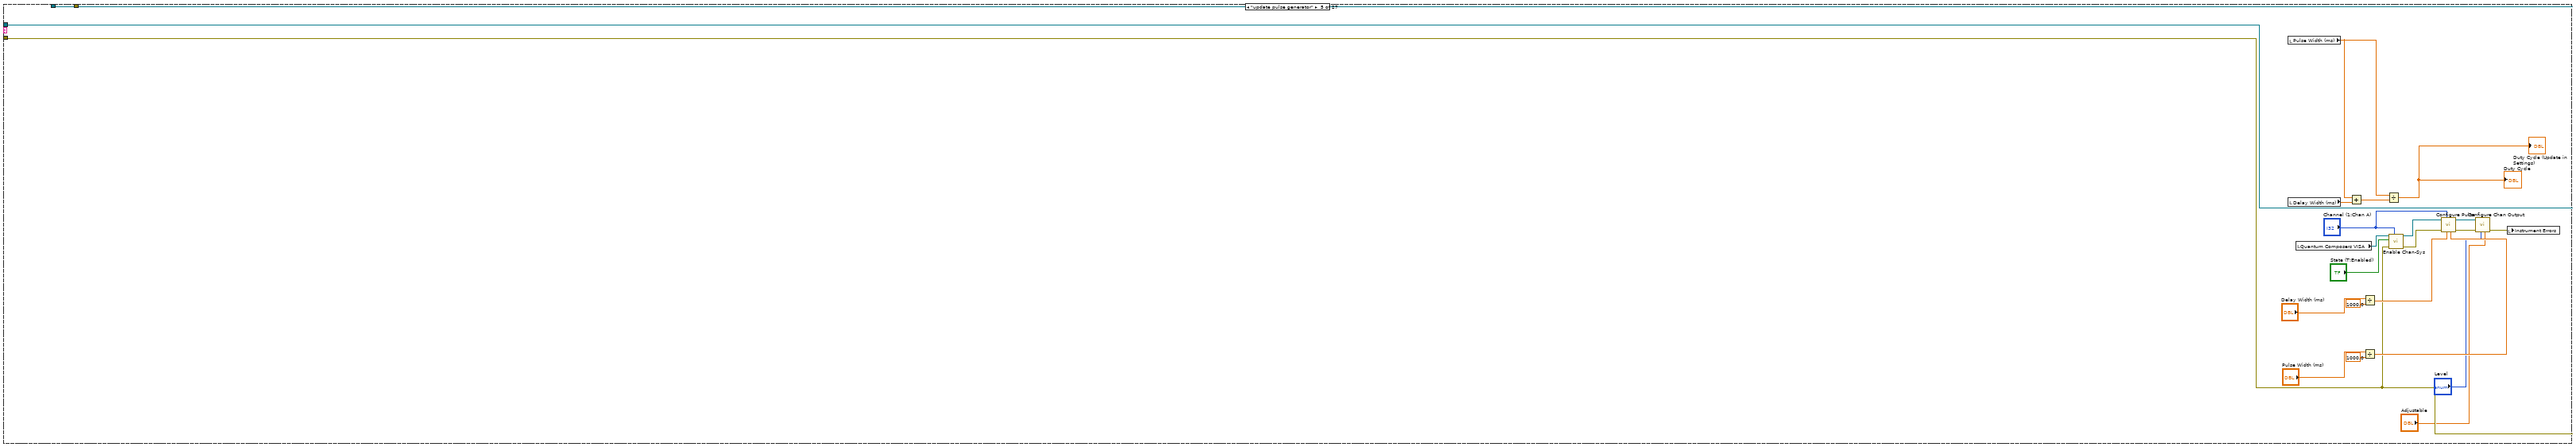
[diagram p9: hidden frame]
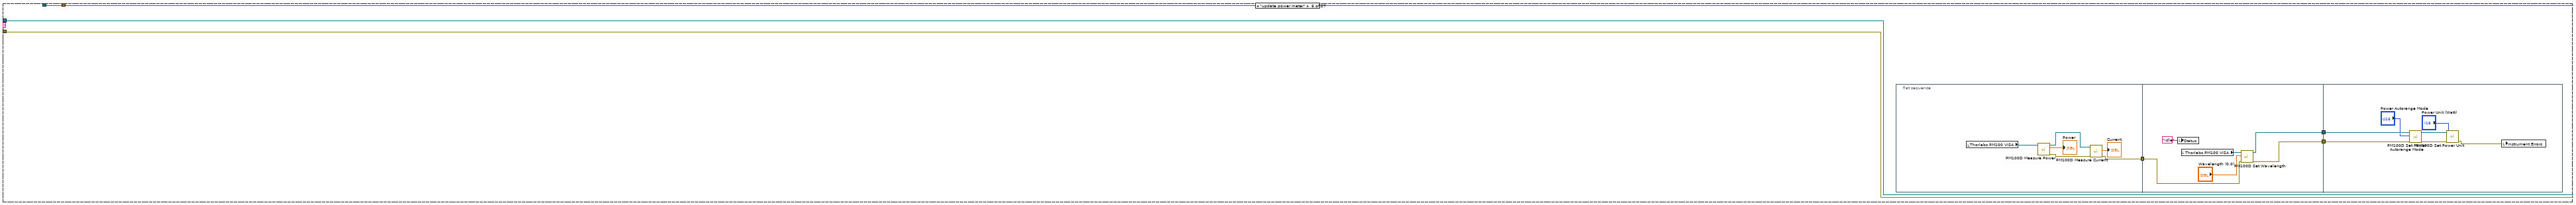
[diagram p10: hidden frame]
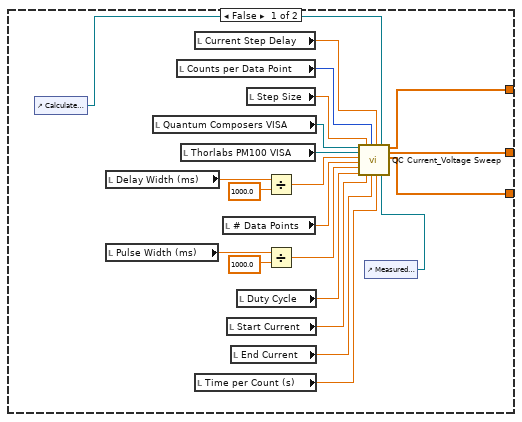
[diagram p12: hidden frame]
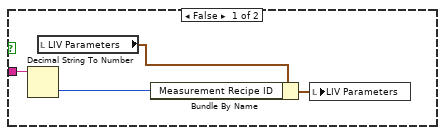
[diagram p13: hidden frame]
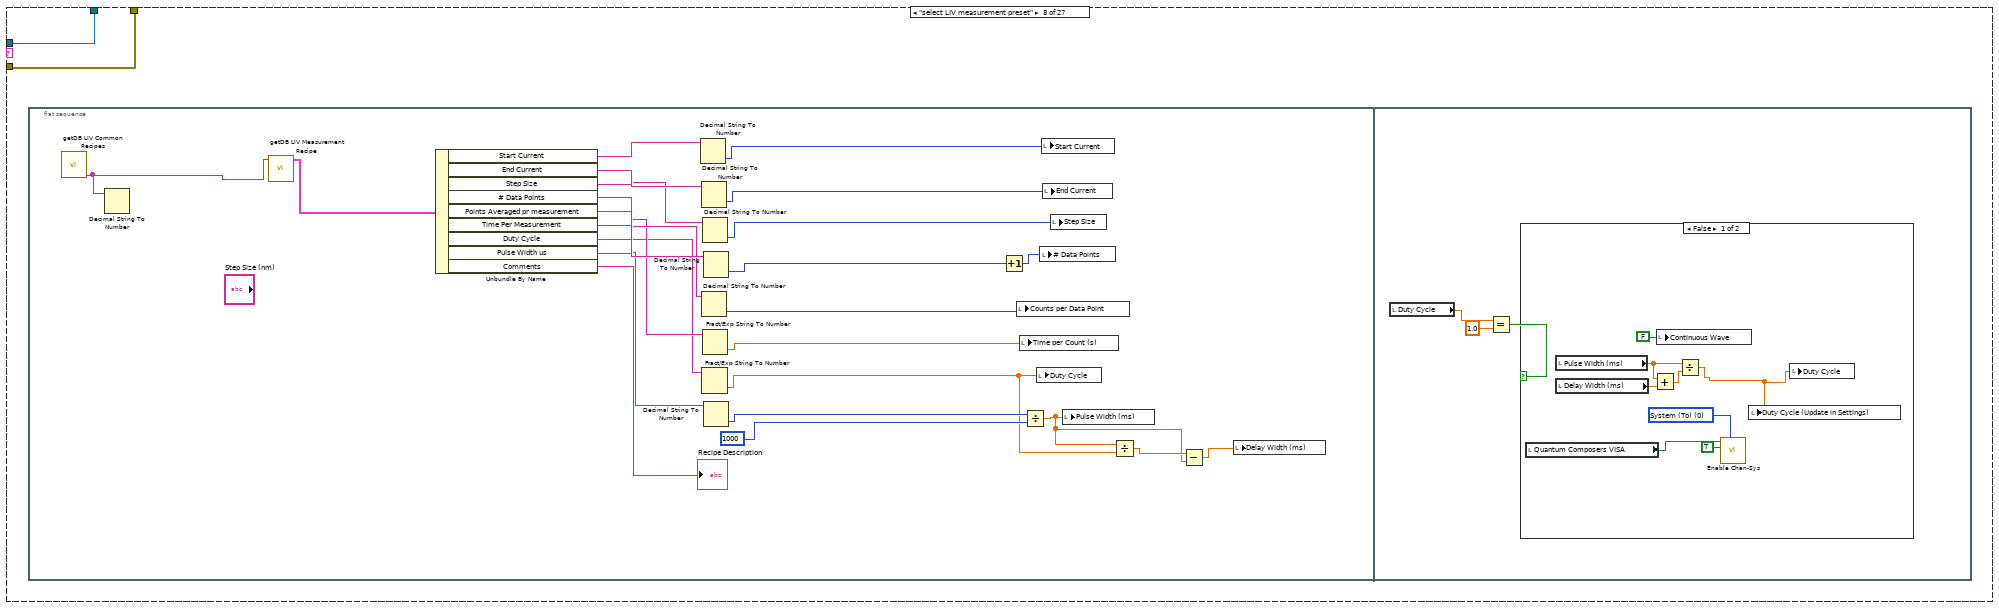
[diagram p14: hidden frame]
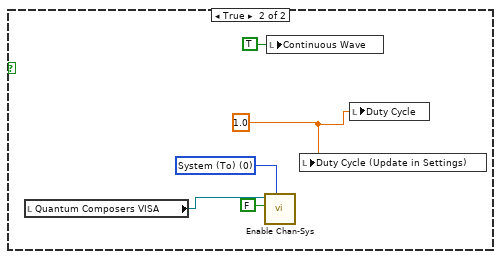
[diagram p15: hidden frame]
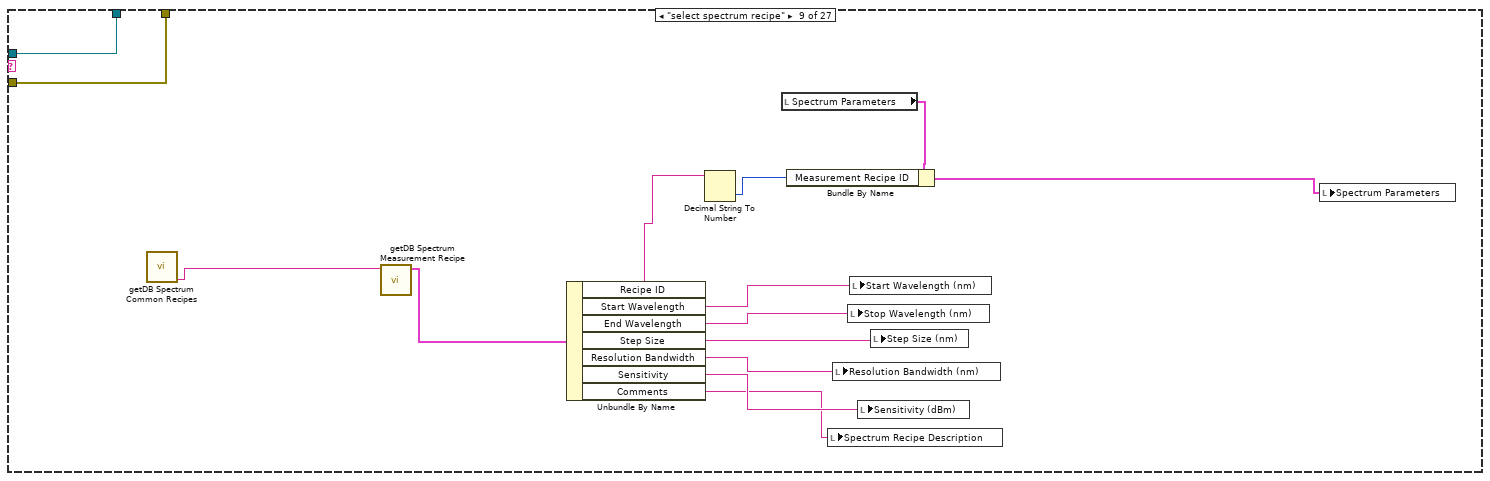
[diagram p16: hidden frame]
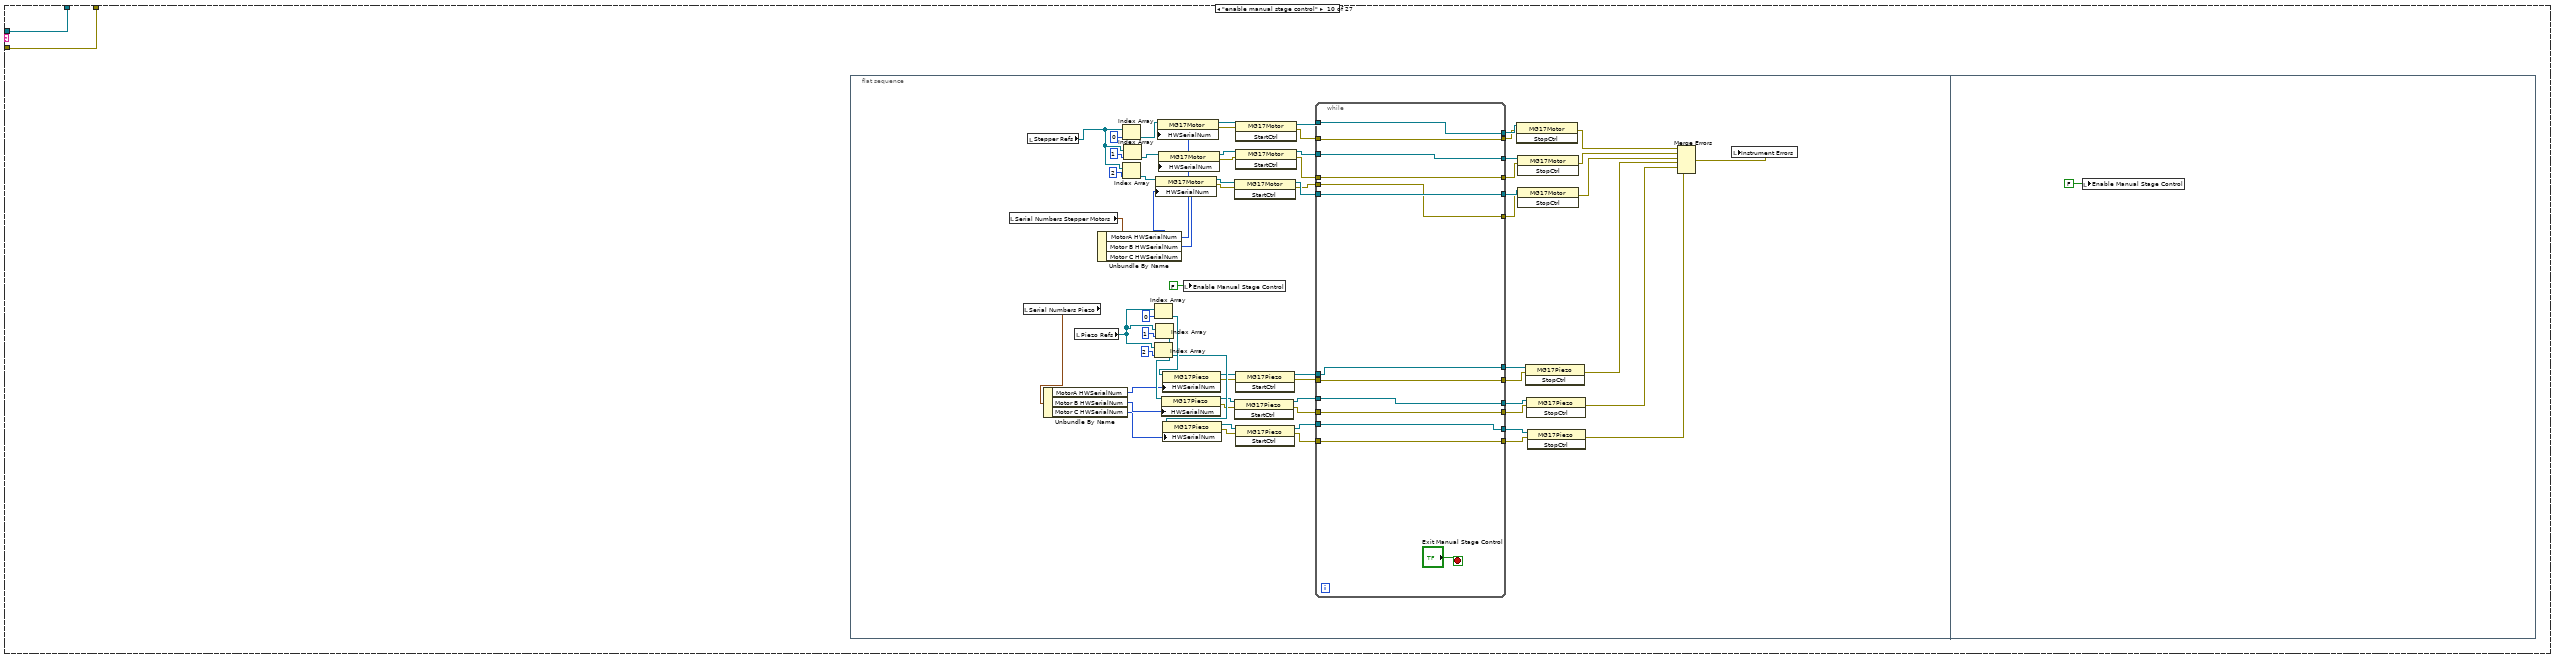
[diagram p17: hidden frame]
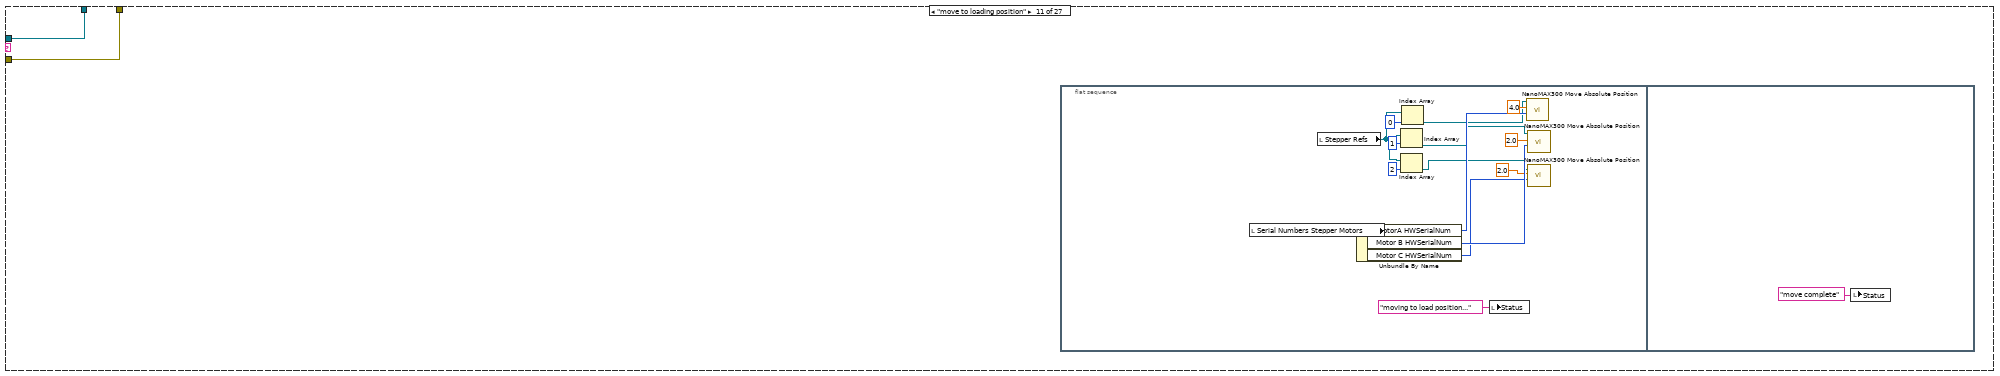
[diagram p18: hidden frame]
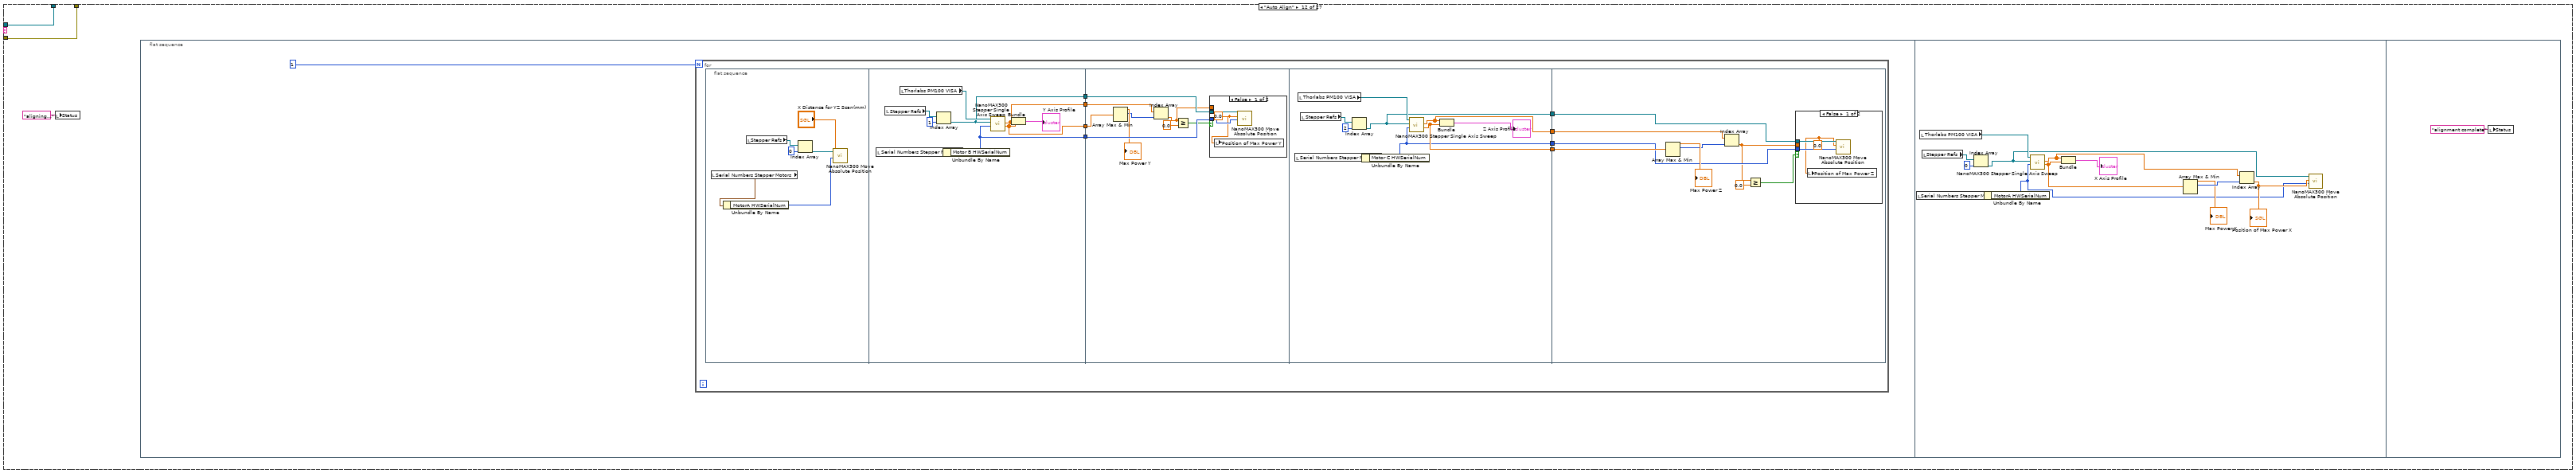
[diagram p19: hidden frame]
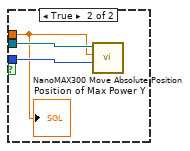
[diagram p20: hidden frame]
diagram:
  n1 = flat-sequence {
    tunnel: [errorcluster {"status"=FALSE, "code"=0, "source"=""} ("error in (no error)")] -> w1
    tunnel: w1 -> [w43]
    frame #0 {
      w24 = errorcluster {"status"=FALSE, "code"=0, "source"=""} ("error in (no error)")
      # "Initialize Instuments"
      n2 = VISA Write(VISA resource name="Agilent OSA Visa", write buffer="*IDN?") -> (VISA resource name out=w8:refnum<visa-resource-name>, return count=w9:u32, error out=w10:errorcluster)  [unwired: 1 in]
      n3 = Build Array("MG17Piezo X Axis", "MG17Piezo Y Axis", "MG17Piezo Z Axis") -> (→"Piezo Refs":refnum<k7>[])
      n4 = VISA Read(VISA resource name=w8, byte count=w9, error in (no error)=w10) -> (read buffer=→"Agilent IDN Query":string, error out=w6:errorcluster)  [unwired: 2 out]
      n5 = call <instrlib>:"Arroyo Initialize.vi"("COM Port"="COM Port") -> ("dup VISA resource name"=→"Arroyo VISA":refnum<visa-resource-name>, "error out"=w27:errorcluster)  [unwired: 3 in]
      n6 = call <instrlib>:"Initialize.vi"("error in (no error)"=w24, "Reset? (T: Yes)"=FALSE, "VISA resource name"="Quantum Composers VISA") -> ("error out"=w23:errorcluster, "VISA resource name out"=w2:refnum<visa-resource-name>)  [unwired: 7 in]
      n7 = call <instrlib>:"PM100D Initialize.vi"("error in (no error)"=w24, "resource name"="Thorlabs PM100 VISA") -> ("error out"=w22:errorcluster)  [unwired: 8 in, 1 out]
      n8 = Open VI Reference(vi path="vi find peak") -> (vi reference=w4:refnum<vi>)  [unwired: 5 in, 1 out]
      n9 = Build Array("Stepper X Axis", "Stepper Y Axis", "Stepper Z Axis") -> (→"Stepper Refs":refnum<k7>[])
      n10 = Merge Errors(w27, w23, w22, w6) -> (→"Instrument Errors":errorcluster)
      n11 = invoke on="Sub Panel" class="SubPanel" method="Insert VI"("VI Ref"=w4) -> ()  [unwired: 3 in, 4 out]
      n12 = call <instrlib>:"Configure Sys (To) Period.vi"("Period (100 msec)"=0.0, "VISA resource name"=w2) -> ()  [unwired: 8 in, 2 out]
    }
    frame #1 {
      w31 = FALSE ("Visible")
      # "Create Variables Here"
      n13 = property on="P array" class="Arr (strict)"("Visible"=w31) -> ()  [unwired: 2 in, 2 out]
      n14 = property on="V Array" class="Arr (strict)"("Visible"=w31) -> ()  [unwired: 2 in, 2 out]
      n15 = property on="I Array" class="Arr (strict)"("Visible"=w31) -> ()  [unwired: 2 in, 2 out]
      "Status" <- "hello" ("Status")
    }
    frame #2 {
      n16 = Obtain Queue(name (unnamed)="q", element data type="test" ("name (unnamed)"), create if not found? (T)=TRUE, error in (no error)=w43) -> (queue out=w35:refnum<queue>, error out=w36:errorcluster)  [unwired: 1 in, 1 out]
      n17 = while {
        shift-right: [w44] -> _
        shift-left: w36 -> [w50]
        shift-right: [w48] -> _
        shift-left: w35 -> [w49]
        stop <- w45 stop-if-true
        n18 = Dequeue Element(queue=w49, error in (no error)=w50) -> (queue out=w47:refnum<queue>, element=w51:string, error out=w46:errorcluster)  [unwired: 1 in, 1 out]
        n19 = case shown="\"update laser driver\"" w51 {
          tunnel: [w53 w56 w59 w60 w108 w113 w137 w294 w348 w350 w432 w451 w553 w556 w603 w712 w730 w752 w764 w766 w783 w803 w806 w811 w813 w1016 w1034] -> w48
          tunnel: w47 -> [w53 w56 w59 w60 w108 w113 w137 w294 w348 w350 w432 w451 w553 w556 w603 w712 w730 w752 w764 w766 w783 w803 w806 w811 w813 w1016 w1034]
          tunnel: [w52 w54 w58 w61 w93 w112 w136 w293 w347 w349 w431 w450 w552 w555 w602 w711 w729 w751 w763 w765 w780 w802 w805 w810 w812 w1015 w1033] -> w44
          tunnel: w46 -> [w52 w54 w58 w61 w93 w112 w136 w293 w347 w349 w431 w450 w552 w555 w602 w711 w729 w751 w763 w765 w780 w802 w805 w810 w812 w1015 w1033]
          tunnel: [_ TRUE _ _ _ _ _ _ _ _ _ _ _ _ _ _ _ _ _ _ _ _ _ _ _ _ _] -> w45
          frame "False", Default {
          }
          frame "stop" {
          }
          frame "idle" {
            n20 = local write "Status"("idle" ("Status")) -> ()
          }
          frame "update laser driver" {
            n21 = flat-sequence {
              frame #0 {
                n22 = case shown="True" "Beep?" {
                  frame False {
                  }
                  frame True {
                    n23 = local read "Arroyo VISA"() -> (w63:refnum<visa-resource-name>)
                    n24 = call <instrlib>:"Arroyo BEEP.vi"("Beep Setting"=i16 2, "VISA resource name"=w63) -> ()  [unwired: 1 in, 2 out]
                  }
                }
              }
              frame #1 {
                n25 = case shown="True" "Laser Output" {
                  selector: "Laser Output" -> [w72 w73]
                  frame False {
                    n26 = local read "COM Port VISA"() -> (w71:refnum<visa-resource-name>)
                    n27 = call <instrlib>:"Arroyo LAS OUTPUT.vi"("Laser Output Enable"=w72, "VISA resource name"=w71) -> ()  [unwired: 1 in, 2 out]
                  }
                  frame True {
                    n28 = call <instrlib>:"Arroyo LAS OUTPUT.vi"("Laser Output Enable"=w73, "VISA resource name"="COM Port VISA") -> ()  [unwired: 1 in, 2 out]
                  }
                }
                n29 = case shown="False" "TEC Output" {
                  selector: "TEC Output" -> [w67 w70]
                  frame False {
                    n30 = local read "COM Port VISA"() -> (w68:refnum<visa-resource-name>)
                    n31 = call <instrlib>:"Arroyo TEC OUTPUT.vi"("TEC Output Enable"=w67, "VISA resource name"=w68) -> ()  [unwired: 1 in, 2 out]
                  }
                  frame True {
                    n32 = local read "COM Port VISA"() -> (w69:refnum<visa-resource-name>)
                    n33 = call <instrlib>:"Arroyo TEC OUTPUT.vi"("TEC Output Enable"=w70, "VISA resource name"=w69) -> ()  [unwired: 1 in, 2 out]
                  }
                }
              }
              frame #2 {
                n34 = local read "Laser Current Setpoint"() -> (w81:dbl)
                n35 = local read "Arroyo VISA"() -> (w76:refnum<visa-resource-name>)
                n36 = Greater Than 0?(x=w81) -> (x > 0?=w80:bool)
                n37 = call <instrlib>:"Arroyo TEC T.vi"("TEC Temperature Setpoint"="TEC Temperature Setpoint", "VISA resource name"=w76) -> ()  [unwired: 1 in, 2 out]
                n38 = call <instrlib>:"Arroyo LAS OUTPUT?.vi"("VISA resource name"=w76) -> ("Laser Output"=w79:bool)  [unwired: 1 in, 2 out]
                n39 = Not(x=w79) -> (.not. x?=w78:bool)
                n40 = And(x=w78, y=w80) -> (x .and. y?=w77:bool)
                n41 = case shown="False" w77 {
                  frame False {
                    n42 = local read "Arroyo VISA"() -> (w82:refnum<visa-resource-name>)
                    n43 = call <instrlib>:"Arroyo LAS LDI.vi"("Laser Current Setpoint"="Laser Current Setpoint", "VISA resource name"=w82) -> ()  [unwired: 1 in, 2 out]
                  }
                  frame True {
                    n44 = call "Display Message to User"() -> ()  [unwired: 10 in, 2 out]
                    n45 = local read "Laser Current Setpoint"() -> (w85:dbl)
                    n46 = local read "Arroyo VISA"() -> (w84:refnum<visa-resource-name>)
                    n47 = call <instrlib>:"Arroyo LAS LDI.vi"("Laser Current Setpoint"=w85, "VISA resource name"=w84) -> ()  [unwired: 1 in, 2 out]
                  }
                }
              }
              frame #3 {
                n48 = local write "Status"("idle" ("Status")) -> ()
              }
            }
          }
          frame "update pulse generator" {
            n49 = local read "Pulse Width (ms)"() -> (w103:dbl)
            n50 = local read "Delay Width (ms)"() -> (w102:dbl)
            n51 = local read "Quantum Composers VISA"() -> (w106:refnum<visa-resource-name>)
            n52 = Add(x=w103, y=w102) -> (x+y=w101:dbl)
            n53 = Divide(x="Delay Width (ms)", y=1000.0) -> (x/y=w98:dbl)
            n54 = Divide(x="Pulse Width (ms)", y=1000.0) -> (x/y=w95:dbl)
            n55 = Divide(x=w103, y=w101) -> (x/y=→"Duty Cycle" →"Duty Cycle (Update in Settings)":dbl)
            n56 = call <instrlib>:"Enable Chan-Sys.vi"("Channel (1:Chan A)"="Channel (1:Chan A)", "error in (no error)"=w93, "State (T:Enabled)"="State (T:Enabled)", "VISA resource name"=w106) -> ("error out"=w92:errorcluster, "VISA resource name out"=w105:refnum<visa-resource-name>)  [unwired: 6 in]
            n57 = call <instrlib>:"Configure Pulse.vi"("Width (10 msec)"=w95, "Delay (10 msec)"=w98, "Channel (1:Chan A)"="Channel (1:Chan A)", "error in (no error)"=w92, "VISA resource name"=w105) -> ("error out"=w91:errorcluster, "VISA resource name out"=w94:refnum<visa-resource-name>)  [unwired: 5 in]
            n58 = call <instrlib>:"Configure Chan Output.vi"("Adjustable (5 Volts)"="Adjustable", "Level (TTL)"="Level", "error in (no error)"=w91, "VISA resource name"=w94) -> ("error out"=w90:errorcluster)  [unwired: 6 in, 1 out]
            n59 = local write "Instrument Errors"(w90) -> ()
          }
          frame "update power meter" {
            n60 = flat-sequence {
              tunnel: [w114] -> w111
              tunnel: w111 -> [w122]
              tunnel: [w121] -> w110
              tunnel: [w120] -> w109
              tunnel: w110 -> [w132]
              tunnel: w109 -> [w128]
              frame #0 {
                n61 = local read "Thorlabs PM100 VISA"() -> (w119:refnum<visa-resource-name>)
                n62 = call <instrlib>:"PM100D Measure Power.vi"("instrument handle"=w119) -> ("error out"=w115:errorcluster, "Power"=→"Power":dbl, "instrument handle out"=w116:refnum<visa-resource-name>)  [unwired: 8 in]
                n63 = call <instrlib>:"PM100D Measure Current.vi"("error in (no error)"=w115, "instrument handle"=w116) -> ("error out"=w114:errorcluster, "Current"=→"Current":dbl)  [unwired: 7 in, 1 out]
              }
              frame #1 {
                n64 = local write "Status"("idle" ("Status")) -> ()
                n65 = local read "Thorlabs PM100 VISA"() -> (w123:refnum<visa-resource-name>)
                n66 = call <instrlib>:"PM100D Set Wavelength.vi"("error in (no error)"=w122, "Wavelength (0.0)"="Wavelength (0.0)", "instrument handle"=w123) -> ("error out"=w120:errorcluster, "instrument handle out"=w121:refnum<visa-resource-name>)  [unwired: 7 in]
              }
              frame #2 {
                n67 = call <instrlib>:"PM100D Set Power Autorange Mode.vi"("error in (no error)"=w128, "Power Autorange Mode (ON)"="Power Autorange Mode", "instrument handle"=w132) -> ("error out"=w127:errorcluster, "instrument handle out"=w131:refnum<visa-resource-name>)  [unwired: 7 in]
                n68 = call <instrlib>:"PM100D Set Power Unit.vi"("error in (no error)"=w127, "Power Unit (Watt)"="Power Unit (Watt)", "instrument handle"=w131) -> ("error out"=w126:errorcluster)  [unwired: 7 in, 1 out]
                n69 = local write "Instrument Errors"(w126) -> ()
              }
            }
          }
          frame "current sweep" {
            n70 = flat-sequence {
              tunnel: [w162] -> w135
              tunnel: [w160] -> w134
              tunnel: [w161] -> w133
              tunnel: w135 -> [w214]
              tunnel: w134 -> [w213]
              tunnel: w133 -> [w212]
              frame #0 {
                n71 = local read "Start Current"() -> (w157:dbl)
                n72 = local read "End Current"() -> (w158:dbl)
                n73 = local read "Arroyo VISA"() -> (w148:refnum<visa-resource-name>)
                n74 = property on="Current Vs. Power" class="XYGraph (strict)"("Value"=cluster{"Y":dbl[], "Y":dbl[]}[] [] ("XY Graph")) -> ()  [unwired: 2 in, 2 out]
                n75 = local write "I Array"(dbl[] [] ("I Array")) -> ()
                n76 = local write "Status"("wait for driver..." ("Status")) -> ()
                n77 = local write "V Array"(dbl[] [] ("V Array")) -> ()
                n78 = local read "Start Current"() -> (w154:dbl)
                "Current Setpoint" <- w154
                n79 = Subtract(x=w158, y=w157) -> (x-y=w156:dbl)
                n80 = call <instrlib>:"Arroyo LAS OUTPUT.vi"("Laser Output Enable"=TRUE, "VISA resource name"=w148) -> ("dup VISA resource name"=w147:refnum<visa-resource-name>)  [unwired: 1 in, 1 out]
                n81 = local read "Counts per Data Point"() -> (w145:i32)
                n82 = call <instrlib>:"Arroyo LAS LDI.vi"("Laser Current Setpoint"=w154, "VISA resource name"=w147) -> ()  [unwired: 1 in, 2 out]
                n83 = local read "Time per Count (s)"() -> (w144:dbl)
                n84 = local read "Step Size"() -> (w155:dbl)
                n85 = Divide(x=w156, y=w155) -> (x/y=w150:dbl)
                n86 = Multiply(x=w145, y=w144) -> (x*y=w143:dbl)
                n87 = Add(x=w150, y=1.0) -> (x+y=w141:dbl)
                "# Data Points" <- w141
                n88 = Add(x=w143, y="Current Step Delay") -> (x+y=w142:dbl)
                n89 = Multiply(x=w141, y=w142) -> (x*y=w140:dbl)
                n90 = local write "Estimated Sweep Time"(w140) -> ()
                n91 = call "Time Delay2"() -> ()  [unwired: 11 in, 1 out]
              }
              frame #1 {
                n92 = local read "Continuous Wave"() -> (w159:bool)
                n93 = local write "Status"("sweeping..." ("Status")) -> ()
                n94 = case shown="True" w159 {
                  tunnel: [w176 w199] -> w162
                  tunnel: [w174 w198] -> w161
                  tunnel: [w175 w197] -> w160
                  frame False {
                    n95 = control-ref of="Calculated Peak Current"() -> (w173:refnum<vi>)
                    n96 = local read "Delay Width (ms)"() -> (w189:dbl)
                    n97 = local read "Pulse Width (ms)"() -> (w187:dbl)
                    n98 = local read "Quantum Composers VISA"() -> (w192:refnum<visa-resource-name>)
                    n99 = local read "Counts per Data Point"() -> (w178:i32)
                    n100 = local read "Thorlabs PM100 VISA"() -> (w191:refnum<visa-resource-name>)
                    n101 = local read "Current Step Delay"() -> (w177:dbl)
                    n102 = local read "Time per Count (s)"() -> (w180:dbl)
                    n103 = local read "# Data Points"() -> (w190:dbl)
                    n104 = local read "Start Current"() -> (w182:dbl)
                    n105 = local read "End Current"() -> (w181:dbl)
                    n106 = local read "Duty Cycle"() -> (w183:dbl)
                    n107 = local read "Step Size"() -> (w179:dbl)
                    n108 = Divide(x=w189, y=1000.0) -> (x/y=w184:dbl)
                    n109 = Divide(x=w187, y=1000.0) -> (x/y=w188:dbl)
                    n110 = control-ref of="Measured Average Current"() -> (w172:refnum<vi>)
                    n111 = call "QC Current_Voltage Sweep.vi"("Quantum Composers VISA"=w192, "Thorlabs PM100 VISA"=w191, "Delay (10 msec)"=w184, "# Data Points"=w190, "Width (10 msec)"=w188, "Duty Cycle"=w183, "Step Size"=w179, "Start Current"=w182, "Counts per Data Point"=w178, "End Current"=w181, "Current Step Time"=w177, "Time per Count (s)"=w180, "Measured Current Ref"=w173, "Peak Current Ref"=w172) -> ("V Array"=w176:dbl[], "I Array"=w175:dbl[], "P Array"=w174:dbl[])  [unwired: 3 in]
                  }
                  frame True {
                    n112 = local read "Counts per Data Point"() -> (w202:i32)
                    n113 = local read "# Data Points"() -> (w200:dbl)
                    n114 = control-ref of="Measured Average Current"() -> (w193:refnum<vi>)
                    n115 = local read "Start Current"() -> (w195:dbl)
                    n116 = local read "Arroyo VISA"() -> (w203:refnum<visa-resource-name>)
                    n117 = local read "End Current"() -> (w196:dbl)
                    n118 = control-ref of="Calculated Peak Current"() -> (w194:refnum<vi>)
                    n119 = local read "Step Size"() -> (w201:dbl)
                    n120 = call "Arroyo Current Sweep.vi"("Arroyo VISA"=w203, "Counts per Data Point"=w202, "Step Size"=w201, "End Current"=w196, "Start Current"=w195, "# Data Points"=w200, "Measured Current Measured Refnum"=w194, "Peak Current Measured Refnum"=w193) -> ("Voltage"=w199:dbl[], "Current"=w197:dbl[], "Power Array"=w198:dbl[])  [unwired: 9 in]
                  }
                }
                "V Array" <- w162
                "I Array" <- w160
                "P array" <- w161
                n121 = call "Time Delay"() -> ()  [unwired: 11 in, 1 out]
                n122 = call "Convert to Dynamic Data3"("Array"=w162) -> ("Dynamic Data Type"=w166:dynamicdata)  [unwired: 3 in]
                n123 = call "Convert to Dynamic Data4"("Array"=w160) -> ("Dynamic Data Type"=w165:dynamicdata)  [unwired: 3 in]
                n124 = call "Convert to Dynamic Data"("Array"=w160) -> ("Dynamic Data Type"=w171:dynamicdata)  [unwired: 3 in]
                n125 = call "Convert to Dynamic Data2"("Array"=w161) -> ("Dynamic Data Type"=w170:dynamicdata)  [unwired: 3 in]
                n126 = call "Build XY Graph2"("Reset"=TRUE, "Y Input"=w165, "X Input"=w166) -> ("XY Graph"=→"Voltage Vs. Current":cluster{"Y":dbl[], "Y":dbl[]}[])  [unwired: 2 in, 6 out]
                n127 = call "Build XY Graph"("Reset"=TRUE, "Y Input"=w170, "X Input"=w171) -> ("XY Graph"=→"Current Vs. Power":cluster{"Y":dbl[], "Y":dbl[]}[])  [unwired: 2 in, 6 out]
              }
              frame #2 {
                n128 = local read "V Array"() -> (w218:dbl[])
                n129 = local read "P array"() -> (w216:dbl[])
                n130 = local read "I Array"() -> (w217:dbl[])
                n131 = call "Caucluate Parameters LIV.vi"("Voltage Array"=w214, "I Array"=w213, "P Array"=w212) -> ("Current @ Max Power"=w204:dbl, "Max Power (mW)"=w211:dbl, "slope efficincy"=w210:dbl, "DQE"=w209:dbl, "energy/photon (eV)"=w208:dbl, "Least Squares Residue"=w207:dbl, "Threshold Voltage (V)"=w205:dbl, "Threshold Current (mA)"=w206:dbl)  [unwired: 5 in]
                n132 = local write "Current @ Max Power"(w204) -> ()
                n133 = local write "Max Power (mW)"(w211) -> ()
                n134 = local write "slope efficincy"(w210) -> ()
                n135 = local write "DQE"(w209) -> ()
                n136 = local write "energy/photon (eV)"(w208) -> ()
                n137 = local write "Least Squares Residue"(w207) -> ()
                n138 = local write "Threshold Current (mA)"(w206) -> ()
                n139 = local write "Threshold Voltage (V)"(w205) -> ()
                n140 = Build Array(w218, w217, w216) -> (w215:dbl[][])
                n141 = local write "LIV Array"(w215) -> ()
              }
              frame #3 {
                n142 = local read "Pulse Width (ms)"() -> (w237:dbl)
                n143 = local read "Temp Setpoint"() -> (w240:string)
                n144 = local read "Arroyo VISA"() -> (w246:refnum<visa-resource-name>)
                n145 = local read "Counts per Data Point"() -> (w232:i32)
                n146 = local read "Time per Count (s)"() -> (w231:dbl)
                n147 = call <instrlib>:"Arroyo LAS OUTPUT.vi"("Laser Output Enable"=FALSE, "VISA resource name"=w246) -> ()  [unwired: 1 in, 2 out]
                n148 = Decimal String To Number(string=w240) -> (number=w244:i32)  [unwired: 2 in, 1 out]
                n149 = local read "Start Current"() -> (w235:dbl)
                n150 = local read "End Current"() -> (w234:dbl)
                n151 = local read "Duty Cycle"() -> (w230:dbl)
                n152 = local read "Step Size"() -> (w233:dbl)
                n153 = Multiply(x=1000.0, y=w237) -> (x*y=w229:dbl)
                n154 = local read "Threshold Current (mA)"() -> (w241:dbl)
                n155 = local read "Threshold Voltage (V)"() -> (w242:dbl)
                n156 = local read "LIV Parameters"() -> (w239:T4)
                n157 = Number To Exponential String(number=w229) -> (E-format string=w222:string)  [unwired: 3 in]
                n158 = Number To Exponential String(number=w235) -> (E-format string=w228:string)  [unwired: 3 in]
                n159 = Number To Exponential String(number=w234) -> (E-format string=w227:string)  [unwired: 3 in]
                n160 = Number To Exponential String(number=w233) -> (E-format string=w226:string)  [unwired: 3 in]
                n161 = Number To Exponential String(number=w232) -> (E-format string=w225:string)  [unwired: 3 in]
                n162 = Number To Exponential String(number=w231) -> (E-format string=w224:string)  [unwired: 3 in]
                n163 = Number To Exponential String(number=w230) -> (E-format string=w223:string)  [unwired: 3 in]
                n164 = local read "DQE"() -> (w243:dbl)
                n165 = Bundle By Name(cluster=w239, "Threshold Current (mA)"=w241, "Threshold Voltage (V)"=w242, "Slope Efficiency"=w243, "Temperature"=w244) -> (w238:T4)
                n166 = call "Check for LIV Measurement Recipe.vi"("pulse width us"=w222, "time per measurement s"=w224, "end current"=w227, "duty cycle"=w223, "points averaged per measurement"=w225, "step size"=w226, "start current"=w228) -> ("Measurement ID"=w219:string)  [unwired: 3 in]
                n167 = local write "LIV Parameters"(w238) -> ()
                n168 = Equal?(x=w219, y="") -> (x = y?=w220:bool)
                n169 = case shown="True" w220 {
                  tunnel: w219 -> [w248 _]
                  frame False {
                    n170 = Decimal String To Number(string=w248) -> (number=w247:i32)  [unwired: 2 in, 1 out]
                    n171 = local read "LIV Parameters"() -> (w250:T4)
                    n172 = Bundle By Name(cluster=w250, "Measurement Recipe ID"=w247) -> (w249:T4)
                    n173 = local write "LIV Parameters"(w249) -> ()
                  }
                  frame True {
                    n174 = local read "Pulse Width (ms)"() -> (w264:dbl)
                    n175 = Multiply(x=1000.0, y=w264) -> (x*y=w272:dbl)
                    n176 = local read "Counts per Data Point"() -> (w269:i32)
                    n177 = local read "Time per Count (s)"() -> (w270:dbl)
                    n178 = local read "# Data Points"() -> (w259:dbl)
                    n179 = local read "Start Current"() -> (w266:dbl)
                    n180 = local read "End Current"() -> (w267:dbl)
                    n181 = local read "Duty Cycle"() -> (w271:dbl)
                    n182 = local read "Step Size"() -> (w268:dbl)
                    n183 = Number To Exponential String(number=w271) -> (E-format string=w256:string)  [unwired: 3 in]
                    n184 = Number To Exponential String(number=w269) -> (E-format string=w257:string)  [unwired: 3 in]
                    n185 = Number To Exponential String(number=w266) -> (E-format string=w263:string)  [unwired: 3 in]
                    n186 = Number To Exponential String(number=w267) -> (E-format string=w262:string)  [unwired: 3 in]
                    n187 = Number To Exponential String(number=w268) -> (E-format string=w261:string)  [unwired: 3 in]
                    n188 = Number To Exponential String(number=w259) -> (E-format string=w260:string)  [unwired: 3 in]
                    n189 = Number To Exponential String(number=w270) -> (E-format string=w258:string)  [unwired: 3 in]
                    n190 = Number To Exponential String(number=w272) -> (E-format string=w251:string)  [unwired: 3 in]
                    n191 = local read "LIV Parameters"() -> (w255:T4)
                    n192 = call "Insert New LIV Recipe into db.vi"("pulse width us"=w251, "duty cycle"=w256, "time per measurement s"=w258, "points averaged per measurement"=w257, "# data points"=w260, "step size"=w261, "end current"=w262, "start current"=w263) -> ("New Measurement ID"=w253:string)  [unwired: 3 in]
                    n193 = Decimal String To Number(string=w253) -> (number=w252:i32)  [unwired: 2 in, 1 out]
                    n194 = Bundle By Name(cluster=w255, "Measurement Recipe ID"=w252) -> (w254:T4)
                    n195 = local write "LIV Parameters"(w254) -> ()
                  }
                }
              }
              frame #4 {
                n196 = flat-sequence {
                  tunnel: [w279] -> w273
                  tunnel: w273 -> [w291]
                  frame #0 {
                    n197 = local read "DeviceInfo"() -> (w278:T2)
                    n198 = local read "WaferInfo"() -> (w281:T5)
                    n199 = local read "Dates"() -> (w276:T1)
                    n200 = Get Date/Time In Seconds() -> (seconds since 1Jan1904=w275:timestamp)
                    n201 = Bundle By Name(cluster=w276, "Measurement Date"=w275) -> (w274:T1)
                    n202 = Unbundle By Name(w281) -> ("WaferName"=w280:string)
                    n203 = Unbundle By Name(w278) -> ("Part Name"=w277:string)
                    n204 = local read "Operator"() -> (w282:string)
                    n205 = local write "Dates"(w274) -> ()
                    n206 = call "get Flash FileName .vi"("Time"=w275, "Device Name"=w277, "Operator"=w282, "Wafer Name"=w280, "FineTest save path"="Sweep save path") -> ("appended path"=w279:path)  [unwired: 6 in]
                  }
                  frame #1 {
                    n207 = local read "LIV Parameters"() -> (w288:T4)
                    n208 = local read "DeviceInfo"() -> (w286:T2)
                    n209 = local read "WaferInfo"() -> (w290:T5)
                    n210 = local read "Operator"() -> (w289:string)
                    n211 = local read "LIV Array"() -> (w287:dbl[][])
                    n212 = local read "Dates"() -> (w284:T1)
                    n213 = call "WriteFlashFile EELS.vi"("Input File Path"=w291, "LIV Parameters"=w288, "LIV Measurement Comments"="LIV Measurement Comments", "Operator"=w289, "WaferInfo"=w290, "Dates"=w284, "DeviceInfo"=w286, "LIV array"=w287) -> ()  [unwired: 7 in, 1 out]
                  }
                }
              }
              frame #5 {
                n214 = local write "Status"("idle" ("Status")) -> ()
              }
            }
          }
          frame "select LIV measurement preset" {
            n215 = flat-sequence {
              frame #0 {
                n216 = call "getDB LIV Common Recipes.vi"() -> ("Desired ID"=w295:string)  [unwired: 11 in]
                n217 = Decimal String To Number(string=w295) -> ()  [unwired: 2 in, 2 out]
                n218 = call "getDB LIV Measurement Recipe.vi"("Recipe ID"=w295) -> ("Recipe Cluster"=w318:T12)  [unwired: 10 in]
                n219 = Unbundle By Name(w318) -> ("Start Current"=w317:string, "End Current"=w316:string, "Step Size"=w313:string, "# Data Points"=w311:string, "Points Averaged pr measurement"=w310:string, "Time Per Measurement"=w301:string, "Duty Cycle"=w299:string, "Pulse Width us"=w308:string, "Comments"=→"Recipe Description":string)
                n220 = Decimal String To Number(string=w317) -> (number=w315:i32)  [unwired: 2 in, 1 out]
                n221 = Decimal String To Number(string=w316) -> (number=w314:i32)  [unwired: 2 in, 1 out]
                n222 = Decimal String To Number(string=w310) -> (number=w309:i32)  [unwired: 2 in, 1 out]
                n223 = Fract/Exp String To Number(string=w299) -> (number=w298:dbl)  [unwired: 3 in, 1 out]
                n224 = Decimal String To Number(string=w313) -> (number=w312:i32)  [unwired: 2 in, 1 out]
                n225 = Fract/Exp String To Number(string=w301) -> (number=w300:dbl)  [unwired: 3 in, 1 out]
                n226 = Decimal String To Number(string=w311) -> (number=w297:i32)  [unwired: 2 in, 1 out]
                n227 = Decimal String To Number(string=w308) -> (number=w307:i32)  [unwired: 2 in, 1 out]
                n228 = Increment(x=w297) -> (x+1=w296:i32)
                n229 = local write "Counts per Data Point"(w309) -> ()
                n230 = local write "Time per Count (s)"(w300) -> ()
                n231 = Divide(x=w307, y=1000) -> (x/y=w303:dbl)
                n232 = local write "Duty Cycle"(w298) -> ()
                n233 = local write "# Data Points"(w296) -> ()
                n234 = local write "Start Current"(w315) -> ()
                n235 = local write "End Current"(w314) -> ()
                n236 = local write "Step Size"(w312) -> ()
                n237 = local write "Pulse Width (ms)"(w303) -> ()
                n238 = Divide(x=w303, y=w298) -> (x/y=w304:dbl)
                n239 = Subtract(x=w304, y=w303) -> (x-y=w302:dbl)
                n240 = local write "Delay Width (ms)"(w302) -> ()
              }
              frame #1 {
                n241 = local read "Duty Cycle"() -> (w321:dbl)
                n242 = Equal?(x=w321, y=1.0) -> (x = y?=w319:bool)
                n243 = case shown="False" w319 {
                  frame False {
                    w328 = 0 items=["System (To)", "Channel A", "Channel B", "Channel C", "Channel D", "Channel E", "Channel F", "Channel G", "Channel H"] ("Channel (1:Chan A)")
                    n244 = local read "Quantum Composers VISA"() -> (w326:refnum<visa-resource-name>)
                    n245 = local read "Pulse Width (ms)"() -> (w323:dbl)
                    n246 = local read "Delay Width (ms)"() -> (w324:dbl)
                    n247 = Add(x=w323, y=w324) -> (x+y=w325:dbl)
                    n248 = local write "Continuous Wave"(FALSE ("Continuous Wave")) -> ()
                    n249 = Divide(x=w323, y=w325) -> (x/y=w322:dbl)
                    n250 = call <instrlib>:"Enable Chan-Sys.vi"("Channel (1:Chan A)"=w328, "State (T:Enabled)"=TRUE, "VISA resource name"=w326) -> ()  [unwired: 7 in, 2 out]
                    n251 = local write "Duty Cycle (Update in Settings)"(w322) -> ()
                    n252 = local write "Duty Cycle"(w322) -> ()
                  }
                  frame True {
                    w333 = 0 items=["System (To)", "Channel A", "Channel B", "Channel C", "Channel D", "Channel E", "Channel F", "Channel G", "Channel H"] ("Channel (1:Chan A)")
                    w330 = 1.0 ("Duty Cycle (Update in Settings)")
                    n253 = local read "Quantum Composers VISA"() -> (w331:refnum<visa-resource-name>)
                    n254 = call <instrlib>:"Enable Chan-Sys.vi"("Channel (1:Chan A)"=w333, "State (T:Enabled)"=FALSE, "VISA resource name"=w331) -> ()  [unwired: 7 in, 2 out]
                    n255 = local write "Continuous Wave"(TRUE ("Continuous Wave")) -> ()
                    n256 = local write "Duty Cycle (Update in Settings)"(w330) -> ()
                    n257 = local write "Duty Cycle"(w330) -> ()
                  }
                }
              }
            }
          }
          frame "select spectrum recipe" {
            n258 = call "getDB Spectrum Common Recipes.vi"() -> ("Desired ID"=w335:string)  [unwired: 11 in]
            n259 = call "getDB Spectrum Measurement Recipe.vi"("Recipe ID"=w335) -> ("Recipe Cluster"=w346:T13)  [unwired: 10 in]
            n260 = Unbundle By Name(w346) -> ("Recipe ID"=w338:string, "Start Wavelength"=w345:string, "End Wavelength"=w344:string, "Step Size"=w343:string, "Resolution Bandwidth"=w342:string, "Sensitivity"=w341:string, "Comments"=w340:string)
            n261 = Decimal String To Number(string=w338) -> (number=w337:i32)  [unwired: 2 in, 1 out]
            n262 = local read "Spectrum Parameters"() -> (w339:T3)
            n263 = Bundle By Name(cluster=w339, "Measurement Recipe ID"=w337) -> (w336:T3)
            n264 = local write "Spectrum Recipe Description"(w340) -> ()
            n265 = local write "Resolution Bandwidth (nm)"(w342) -> ()
            n266 = local write "Stop Wavelength (nm)"(w344) -> ()
            n267 = local write "Start Wavelength (nm)"(w345) -> ()
            n268 = local write "Sensitivity (dBm)"(w341) -> ()
            n269 = local write "Step Size (nm)"(w343) -> ()
            n270 = local write "Spectrum Parameters"(w336) -> ()
          }
          frame "enable manual stage control" {
            n271 = flat-sequence {
              frame #0 {
                n272 = local read "Serial Numbers Stepper Motors"() -> (w415:T10)
                n273 = local read "Serial Numbers Piezo"() -> (w404:T10)
                n274 = local read "Stepper Refs"() -> (w410:refnum<k7>[])
                n275 = Unbundle By Name(w404) -> ("MotorA HWSerialNum"=w376:i32, "Motor B HWSerialNum"=w403:i32, "Motor C HWSerialNum"=w402:i32)
                n276 = local read "Piezo Refs"() -> (w396:refnum<k7>[])
                n277 = Unbundle By Name(w415) -> ("MotorA HWSerialNum"=w413:i32, "Motor B HWSerialNum"=w408:i32, "Motor C HWSerialNum"=w406:i32)
                n278 = Index Array(array=w410, index=0) -> (element=w414:refnum<k7>)
                n279 = Index Array(array=w410, index=2) -> (element=w407:refnum<k7>)
                n280 = Index Array(array=w410, index=1) -> (element=w409:refnum<k7>)
                n281 = Index Array(array=w396, index=0) -> (element=w398:refnum<k7>)
                n282 = Index Array(array=w396, index=2) -> (element=w395:refnum<k7>)
                n283 = property class="MG17Motor"(reference=w407, "HWSerialNum"=w406) -> (reference out=w371:refnum<k7>, error out=w368:errorcluster)  [unwired: 1 in]
                n284 = Index Array(array=w396, index=1) -> (element=w397:refnum<k7>)
                n285 = property class="MG17Motor"(reference=w414, "HWSerialNum"=w413) -> (reference out=w375:refnum<k7>, error out=w365:errorcluster)  [unwired: 1 in]
                n286 = property class="MG17Motor"(reference=w409, "HWSerialNum"=w408) -> (reference out=w373:refnum<k7>, error out=w366:errorcluster)  [unwired: 1 in]
                n287 = property class="MG17Piezo"(reference=w397, "HWSerialNum"=w403) -> (reference out=w359:refnum<k7>, error out=w362:errorcluster)  [unwired: 1 in]
                n288 = property class="MG17Piezo"(reference=w398, "HWSerialNum"=w376) -> (reference out=w358:refnum<k7>, error out=w363:errorcluster)  [unwired: 1 in]
                n289 = property class="MG17Piezo"(reference=w395, "HWSerialNum"=w402) -> (reference out=w360:refnum<k7>, error out=w361:errorcluster)  [unwired: 1 in]
                n290 = local write "Enable Manual Stage Control"(FALSE ("Enable Manual Stage Control")) -> ()
                n291 = invoke class="MG17Motor" method="StartCtrl"(reference=w371, error in=w368) -> (reference out=w370:refnum<k7>, error out=w369:errorcluster)  [unwired: 1 in, 1 out]
                n292 = invoke class="MG17Piezo" method="StartCtrl"(reference=w359, error in=w362) -> (reference out=w355:refnum<k7>, error out=w354:errorcluster)  [unwired: 1 in, 1 out]
                n293 = invoke class="MG17Motor" method="StartCtrl"(reference=w375, error in=w365) -> (reference out=w374:refnum<k7>, error out=w364:errorcluster)  [unwired: 1 in, 1 out]
                n294 = invoke class="MG17Motor" method="StartCtrl"(reference=w373, error in=w366) -> (reference out=w372:refnum<k7>, error out=w367:errorcluster)  [unwired: 1 in, 1 out]
                n295 = invoke class="MG17Piezo" method="StartCtrl"(reference=w358, error in=w363) -> (reference out=w357:refnum<k7>, error out=w356:errorcluster)  [unwired: 1 in, 1 out]
                n296 = invoke class="MG17Piezo" method="StartCtrl"(reference=w360, error in=w361) -> (reference out=w353:refnum<k7>, error out=w352:errorcluster)  [unwired: 1 in, 1 out]
                n297 = while {
                  tunnel: w357 -> [w428]
                  tunnel: [w428] -> w394
                  tunnel: [w427] -> w393
                  tunnel: w355 -> [w427]
                  tunnel: [w426] -> w392
                  tunnel: w353 -> [w426]
                  tunnel: [w425] -> w391
                  tunnel: w356 -> [w425]
                  tunnel: [w424] -> w390
                  tunnel: w354 -> [w424]
                  tunnel: [w423] -> w389
                  tunnel: w352 -> [w423]
                  tunnel: [w422] -> w385
                  tunnel: w374 -> [w422]
                  tunnel: w364 -> [w421]
                  tunnel: [w421] -> w384
                  tunnel: [w420] -> w383
                  tunnel: w372 -> [w420]
                  tunnel: [w419] -> w382
                  tunnel: w367 -> [w419]
                  tunnel: [w418] -> w381
                  tunnel: w370 -> [w418]
                  tunnel: [w417] -> w380
                  tunnel: w369 -> [w417]
                  stop <- "Exit Manual Stage Control" stop-if-true
                }
                n298 = invoke class="MG17Motor" method="StopCtrl"(reference=w385, error in=w384) -> (error out=w379:errorcluster)  [unwired: 1 in, 2 out]
                n299 = invoke class="MG17Motor" method="StopCtrl"(reference=w383, error in=w382) -> (error out=w378:errorcluster)  [unwired: 1 in, 2 out]
                n300 = invoke class="MG17Motor" method="StopCtrl"(reference=w381, error in=w380) -> (error out=w377:errorcluster)  [unwired: 1 in, 2 out]
                n301 = invoke class="MG17Piezo" method="StopCtrl"(reference=w394, error in=w391) -> (error out=w388:errorcluster)  [unwired: 1 in, 2 out]
                n302 = invoke class="MG17Piezo" method="StopCtrl"(reference=w393, error in=w390) -> (error out=w387:errorcluster)  [unwired: 1 in, 2 out]
                n303 = invoke class="MG17Piezo" method="StopCtrl"(reference=w392, error in=w389) -> (error out=w386:errorcluster)  [unwired: 1 in, 2 out]
                n304 = Merge Errors(w379, w378, w377, w388, w387, w386) -> (w405:errorcluster)
                n305 = local write "Instrument Errors"(w405) -> ()
              }
              frame #1 {
                n306 = local write "Enable Manual Stage Control"(FALSE ("Enable Manual Stage Control")) -> ()
              }
            }
          }
          frame "move to loading position" {
            n307 = flat-sequence {
              frame #0 {
                n308 = local read "Serial Numbers Stepper Motors"() -> (w443:T10)
                n309 = local read "Stepper Refs"() -> (w447:refnum<k7>[])
                n310 = Unbundle By Name(w443) -> ("MotorA HWSerialNum"=w442:i32, "Motor B HWSerialNum"=w441:i32, "Motor C HWSerialNum"=w440:i32)
                n311 = Index Array(array=w447, index=1) -> (element=w435:refnum<k7>)
                n312 = Index Array(array=w447, index=2) -> (element=w434:refnum<k7>)
                n313 = Index Array(array=w447, index=0) -> (element=w436:refnum<k7>)
                n314 = local write "Status"("moving to load position..." ("Status")) -> ()
                n315 = call "NanoMAX300 Move Absolute Position.vi"("Serial number"=w442, "Move Postion"=sgl 4.0, "Automation Refnum in"=w436) -> ()  [unwired: 9 in]
                n316 = call "NanoMAX300 Move Absolute Position.vi"("Serial number"=w441, "Move Postion"=sgl 2.0, "Automation Refnum in"=w435) -> ()  [unwired: 9 in]
                n317 = call "NanoMAX300 Move Absolute Position.vi"("Serial number"=w440, "Move Postion"=sgl 2.0, "Automation Refnum in"=w434) -> ()  [unwired: 9 in]
              }
              frame #1 {
                n318 = local write "Status"("move complete" ("Status")) -> ()
              }
            }
          }
          frame "Auto Align" {
            n319 = local write "Status"("aligning..." ("Status")) -> ()
            n320 = flat-sequence {
              frame #0 {
                n321 = for {
                  N: 1 -> [_]
                  n322 = flat-sequence {
                    tunnel: [w470] -> w460
                    tunnel: [w469] -> w459
                    tunnel: [w468] -> w458
                    tunnel: [w467] -> w457
                    tunnel: w460 -> [w484]
                    tunnel: w459 -> [w483]
                    tunnel: w458 -> [w482]
                    tunnel: w457 -> [w481]
                    tunnel: [w494] -> w456
                    tunnel: [w493] -> w455
                    tunnel: [w492] -> w454
                    tunnel: [w491] -> w453
                    tunnel: w456 -> [w506]
                    tunnel: w455 -> [w505]
                    tunnel: w454 -> [w504]
                    tunnel: w453 -> [w503]
                    frame #0 {
                      n323 = local read "Serial Numbers Stepper Motors"() -> (w463:T10)
                      n324 = Unbundle By Name(w463) -> ("MotorA HWSerialNum"=w462:i32)
                      n325 = local read "Stepper Refs"() -> (w465:refnum<k7>[])
                      n326 = Index Array(array=w465, index=0) -> (element=w464:refnum<k7>)
                      n327 = call "NanoMAX300 Move Absolute Position.vi"("Serial number"=w462, "Move Postion"="X Distance for YZ Scan(mm)", "Automation Refnum in"=w464) -> ()  [unwired: 9 in]
                    }
                    frame #1 {
                      n328 = local read "Serial Numbers Stepper Motors"() -> (w473:T10)
                      n329 = local read "Stepper Refs"() -> (w475:refnum<k7>[])
                      n330 = local read "Thorlabs PM100 VISA"() -> (w471:refnum<visa-resource-name>)
                      n331 = Index Array(array=w475, index=1) -> (element=w467:refnum<k7>)
                      n332 = Unbundle By Name(w473) -> ("Motor B HWSerialNum"=w468:i32)
                      n333 = call "NanoMAX300 Stepper Single Axis Sweep.vi"("MotorA HWSerialNum"=w468, "stepper"=w467, "PM100 Visa"=w471) -> ("Power Array"=w470:dbl[], "Position Array"=w469:sgl[])  [unwired: 6 in]
                      n334 = Bundle("Position Array"=w469, "Power Array"=w470) -> (→"Y Axis Profile":T9)  [unwired: 1 in]
                    }
                    frame #2 {
                      n335 = Array Max & Min(array=w484) -> (max value=→"Max Power Y":dbl, max index (indices)=w479:i32)  [unwired: 2 out]
                      n336 = Index Array(array=w483, index=w479) -> (element=w476:sgl)
                      n337 = Greater Or Equal?(x=w476, y=sgl 0.0) -> (x >= y?=w477:bool)
                      n338 = case shown="False" w477 {
                        tunnel: w482 -> [w486 w490]
                        tunnel: w481 -> [w487 w489]
                        tunnel: w476 -> [_ w488]
                        frame False {
                          w485 = sgl 0.0 ("Move Postion")
                          n339 = local write "Position of Max Power Y"(w485) -> ()
                          n340 = call "NanoMAX300 Move Absolute Position.vi"("Serial number"=w486, "Move Postion"=w485, "Automation Refnum in"=w487) -> ()  [unwired: 9 in]
                        }
                        frame True {
                          n341 = call "NanoMAX300 Move Absolute Position.vi"("Serial number"=w490, "Move Postion"=w488, "Automation Refnum in"=w489) -> ()  [unwired: 9 in]
                          "Position of Max Power Y" <- w488
                        }
                      }
                    }
                    frame #3 {
                      n342 = local read "Serial Numbers Stepper Motors"() -> (w497:T10)
                      n343 = local read "Thorlabs PM100 VISA"() -> (w496:refnum<visa-resource-name>)
                      n344 = local read "Stepper Refs"() -> (w498:refnum<k7>[])
                      n345 = Index Array(array=w498, index=2) -> (element=w492:refnum<k7>)
                      n346 = Unbundle By Name(w497) -> ("Motor C HWSerialNum"=w491:i32)
                      n347 = call "NanoMAX300 Stepper Single Axis Sweep.vi"("MotorA HWSerialNum"=w491, "stepper"=w492, "PM100 Visa"=w496) -> ("Power Array"=w494:dbl[], "Position Array"=w493:sgl[])  [unwired: 6 in]
                      n348 = Bundle("Position Array"=w493, "Power Array"=w494) -> (→"Z Axis Profile":T9)  [unwired: 1 in]
                    }
                    frame #4 {
                      n349 = Array Max & Min(array=w506) -> (max value=→"Max Power Z":dbl, max index (indices)=w507:i32)  [unwired: 2 out]
                      n350 = Index Array(array=w505, index=w507) -> (element=w500:sgl)
                      n351 = Greater Or Equal?(x=w500, y=sgl 0.0) -> (x >= y?=w501:bool)
                      n352 = case shown="False" w501 {
                        tunnel: w500 -> [_ w512]
                        tunnel: w504 -> [w511 w514]
                        tunnel: w503 -> [w510 w513]
                        frame False {
                          w509 = sgl 0.0 ("y")
                          n353 = local write "Position of Max Power Z"(w509) -> ()
                          n354 = call "NanoMAX300 Move Absolute Position.vi"("Serial number"=w510, "Move Postion"=w509, "Automation Refnum in"=w511) -> ()  [unwired: 9 in]
                        }
                        frame True {
                          n355 = call "NanoMAX300 Move Absolute Position.vi"("Serial number"=w513, "Move Postion"=w512, "Automation Refnum in"=w514) -> ()  [unwired: 9 in]
                          "Position of Max Power Z" <- w512
                        }
                      }
                    }
                  }
                }
              }
              frame #1 {
                n356 = local read "Serial Numbers Stepper Motors"() -> (w521:T10)
                n357 = local read "Thorlabs PM100 VISA"() -> (w522:refnum<visa-resource-name>)
                n358 = local read "Stepper Refs"() -> (w520:refnum<k7>[])
                n359 = Index Array(array=w520, index=0) -> (element=w516:refnum<k7>)
                n360 = Unbundle By Name(w521) -> ("MotorA HWSerialNum"=w515:i32)
                n361 = call "NanoMAX300 Stepper Single Axis Sweep.vi"("MotorA HWSerialNum"=w515, "stepper"=w516, "PM100 Visa"=w522) -> ("Power Array"=w517:dbl[], "Position Array"=w518:sgl[])  [unwired: 6 in]
                n362 = Bundle("Position Array"=w518, "Power Array"=w517) -> (→"X Axis Profile":T9)  [unwired: 1 in]
                n363 = Array Max & Min(array=w517) -> (max value=→"Max Power X":dbl, max index (indices)=w525:i32)  [unwired: 2 out]
                n364 = Index Array(array=w518, index=w525) -> (element=w526:sgl)
                "Position of Max Power X" <- w526
                n365 = call "NanoMAX300 Move Absolute Position.vi"("Serial number"=w515, "Move Postion"=w526, "Automation Refnum in"=w516) -> ()  [unwired: 9 in]
              }
              frame #2 {
                n366 = local write "Status"("alignment complete" ("Status")) -> ()
              }
            }
          }
          frame "osa settings update" {
            n367 = local read "Agilent OSA Visa"() -> (w551:refnum<visa-resource-name>)
            n368 = Concatenate Strings("sens:wav:star " ("string"), "Start Wavelength (nm)", "nm" ("string")) -> (w547:string)
            n369 = VISA Write(VISA resource name=w551, write buffer=w547) -> (VISA resource name out=w545:refnum<visa-resource-name>, error out=w546:errorcluster)  [unwired: 1 in, 1 out]
            n370 = Concatenate Strings("sens:wav:stop " ("string"), "Stop Wavelength (nm)", "nm" ("string")) -> (w541:string)
            n371 = VISA Write(VISA resource name=w545, write buffer=w541, error in (no error)=w546) -> (VISA resource name out=w540:refnum<visa-resource-name>, error out=w534:errorcluster)  [unwired: 1 out]
            n372 = Concatenate Strings("sens:pow:dc:rang:low " ("string"), "Sensitivity (dBm)", "dBm" ("string")) -> (w536:string)
            n373 = VISA Write(VISA resource name=w540, write buffer=w536, error in (no error)=w534) -> (VISA resource name out=w535:refnum<visa-resource-name>, error out=w533:errorcluster)  [unwired: 1 out]
            n374 = Concatenate Strings("sens:bwid:res " ("string"), "Resolution Bandwidth (nm)", "nm" ("string")) -> (w529:string)
            n375 = VISA Write(VISA resource name=w535, write buffer=w529, error in (no error)=w533) -> (error out=w528:errorcluster)  [unwired: 2 out]
            n376 = local write "OSA Error"(w528) -> ()
          }
          frame "save OSA spectrum" {
            n377 = flat-sequence {
              tunnel: [w580] -> w554
              tunnel: w554 -> [w590]
              frame #0 {
                n378 = local read "Resolution Bandwidth (nm)"() -> (w560:string)
                n379 = local read "Start Wavelength (nm)"() -> (w564:string)
                n380 = local read "Stop Wavelength (nm)"() -> (w563:string)
                n381 = local read "Step Size (nm)"() -> (w562:string)
                n382 = local read "Sensitivity (dBm)"() -> (w561:string)
                n383 = call "Check for Spectrum Measurement Recipe.vi"("sensitivity"=w561, "end wavelenth"=w563, "resolution bandwidth"=w560, "step size"=w562, "start wavelength"=w564) -> ("Measurement ID"=w557:string)  [unwired: 5 in]
                n384 = Equal?(x=w557, y="") -> (x = y?=w558:bool)
                n385 = case shown="True" w558 {
                  tunnel: w557 -> [w566 _]
                  frame False {
                    n386 = Decimal String To Number(string=w566) -> (number=w565:i32)  [unwired: 2 in, 1 out]
                    n387 = local read "Spectrum Parameters"() -> (w568:T3)
                    n388 = Bundle By Name(cluster=w568, "Measurement Recipe ID"=w565) -> (w567:T3)
                    n389 = local write "Spectrum Parameters"(w567) -> ()
                  }
                  frame True {
                    n390 = local read "Resolution Bandwidth (nm)"() -> (w574:string)
                    n391 = local read "Start Wavelength (nm)"() -> (w577:string)
                    n392 = local read "Stop Wavelength (nm)"() -> (w576:string)
                    n393 = local read "Step Size (nm)"() -> (w575:string)
                    n394 = local read "Sensitivity (dBm)"() -> (w573:string)
                    n395 = call "Insert New Spectrum Recipe into db.vi"("sensitivity"=w573, "resolution bandwidth"=w574, "step size"=w575, "end wavelength"=w576, "start wavelength"=w577) -> ("New Measurement ID"=w571:string)  [unwired: 6 in]
                    n396 = Decimal String To Number(string=w571) -> (number=w570:i32)  [unwired: 2 in, 1 out]
                    n397 = local read "Spectrum Parameters"() -> (w572:T3)
                    n398 = Bundle By Name(cluster=w572, "Measurement Recipe ID"=w570) -> (w569:T3)
                    n399 = local write "Spectrum Parameters"(w569) -> ()
                  }
                }
              }
              frame #1 {
                n400 = local read "WaferInfo"() -> (w584:T5)
                n401 = local read "Operator"() -> (w582:string)
                n402 = local read "DeviceInfo"() -> (w579:T2)
                n403 = Unbundle By Name(w584) -> ("WaferName"=w583:string)
                n404 = Unbundle By Name(w579) -> ("Part Name"=w578:string)
                n405 = Get Date/Time In Seconds() -> (seconds since 1Jan1904=w581:timestamp)
                n406 = call "get Spectrum FileName.vi"("Time"=w581, "Device Name"=w578, "Operator"=w582, "Wafer Name"=w583, "FineTest save path"="Spectrum File Location") -> ("appended path"=w580:path)  [unwired: 6 in]
              }
              frame #2 {
                n407 = local read "DeviceInfo"() -> (w589:T2)
                n408 = local read "WaferInfo"() -> (w591:T5)
                n409 = local read "Dates"() -> (w587:T1)
                n410 = local read "Wavelength Array"() -> (w593:dbl[])
                n411 = Unbundle By Name(w589) -> ("Part Name"=w588:string)
                n412 = local read "intensity array"() -> (w594:dbl[])
                n413 = local read "Operator"() -> (w596:string)
                n414 = Build Array(w593, w594) -> (w592:dbl[][])
                n415 = local read "Spectrum Parameters"() -> (w595:T3)
                n416 = call "WriteFlashFile Spectrum.vi"("Input File Path"=w590, "Spectrum Parameters"=w595, "Operator"=w596, "WaferInfo"=w591, "Dates"=w587, "Device Name"=w588, "Spectrum array"=w592, "Comments"="Comments on Spectrum") -> ()  [unwired: 7 in, 1 out]
              }
            }
          }
          frame "osa sweep" {
            n417 = flat-sequence {
              tunnel: [w632] -> w601
              tunnel: [w625] -> w600
              tunnel: [w624] -> w599
              tunnel: w601 -> [w682]
              tunnel: w600 -> [w683]
              tunnel: w599 -> [w681]
              tunnel: [w681] -> w598
              tunnel: [w680] -> w597
              tunnel: w598 -> [w707]
              tunnel: w597 -> [w706]
              frame #0 {
                n418 = local read "Agilent OSA Visa"() -> (w666:refnum<visa-resource-name>)
                n419 = VISA Write(VISA resource name=w666, write buffer="init:imm") -> (VISA resource name out=w664:refnum<visa-resource-name>, error out=w663:errorcluster)  [unwired: 1 in, 1 out]
                n420 = while {
                  tunnel: w664 -> [w679]
                  tunnel: w663 -> [w678]
                  tunnel: [w673] -> w662
                  tunnel: [w672] -> w660
                  stop <- w674 stop-if-true
                  n421 = VISA Write(VISA resource name=w679, write buffer="*opc?", error in (no error)=w678) -> (VISA resource name out=w677:refnum<visa-resource-name>, return count=w675:u32, error out=w676:errorcluster)
                  n422 = Wait (ms)(milliseconds to wait=u32 250) -> ()  [unwired: 1 out]
                  n423 = VISA Read(VISA resource name=w677, byte count=w675, error in (no error)=w676) -> (VISA resource name out=w673:refnum<visa-resource-name>, read buffer=w669:string, error out=w672:errorcluster)  [unwired: 1 out]
                  n424 = Decimal String To Number(string=w669) -> (number=w668:i32)  [unwired: 2 in, 1 out]
                  n425 = Equal?(x=w668, y=1) -> (x = y?=w674:bool)
                }
                n426 = VISA Write(VISA resource name=w662, write buffer="calc1:mark1:max", error in (no error)=w660) -> (VISA resource name out=w659:refnum<visa-resource-name>, error out=w656:errorcluster)  [unwired: 1 out]
                n427 = VISA Write(VISA resource name=w659, write buffer="calc1:mark1:x?", error in (no error)=w656) -> (VISA resource name out=w658:refnum<visa-resource-name>, return count=w657:u32, error out=w655:errorcluster)
                n428 = VISA Read(VISA resource name=w658, byte count=w657, error in (no error)=w655) -> (VISA resource name out=w653:refnum<visa-resource-name>, read buffer=w608:string, error out=w652:errorcluster)  [unwired: 1 out]
                n429 = Fract/Exp String To Number(string=w608) -> (number=w607:dbl)  [unwired: 3 in, 1 out]
                n430 = VISA Write(VISA resource name=w653, write buffer="calc1:mark1:y?", error in (no error)=w652) -> (VISA resource name out=w650:refnum<visa-resource-name>, return count=w648:u32, error out=w649:errorcluster)
                n431 = Multiply(x=w607, y=1000.0) -> (x*y=w604:dbl)
                n432 = Number To Exponential String(number=w604) -> (E-format string=→"Peak Wavelength (nm)":string)  [unwired: 3 in]
                n433 = VISA Read(VISA resource name=w650, byte count=w648, error in (no error)=w649) -> (VISA resource name out=w615:refnum<visa-resource-name>, read buffer=→"Peak Intensity (dBm)":string, error out=w616:errorcluster)  [unwired: 1 out]
                n434 = VISA Write(VISA resource name=w615, write buffer="calc1:mark1:func:bwid:read w", error in (no error)=w616) -> (VISA resource name out=w622:refnum<visa-resource-name>, error out=w623:errorcluster)  [unwired: 1 out]
                n435 = VISA Write(VISA resource name=w622, write buffer="calc1:mark1:func:bwid:stat on", error in (no error)=w623) -> (VISA resource name out=w620:refnum<visa-resource-name>, error out=w621:errorcluster)  [unwired: 1 out]
                n436 = VISA Write(VISA resource name=w620, write buffer="calc1:mark1:func:bwid:res?", error in (no error)=w621) -> (VISA resource name out=w617:refnum<visa-resource-name>, return count=w618:u32, error out=w619:errorcluster)
                n437 = VISA Read(VISA resource name=w617, byte count=w618, error in (no error)=w619) -> (VISA resource name out=w614:refnum<visa-resource-name>, read buffer=w609:string, error out=w613:errorcluster)  [unwired: 1 out]
                n438 = local write "FWHM (nm)"(w609) -> ()
                n439 = VISA Write(VISA resource name=w614, write buffer="form ascii", error in (no error)=w613) -> (VISA resource name out=w643:refnum<visa-resource-name>, error out=w644:errorcluster)  [unwired: 1 out]
                n440 = VISA Write(VISA resource name=w643, write buffer="trac:data:y? tra", error in (no error)=w644) -> (VISA resource name out=w642:refnum<visa-resource-name>)  [unwired: 2 out]
                n441 = VISA Read(VISA resource name=w642, byte count="byte count") -> (read buffer=w639:string, error out=→"OSA Error":errorcluster)  [unwired: 1 in, 2 out]
                n442 = Spreadsheet String To Array(delimiter (Tab)=",", format string="%f", spreadsheet string=w639, array type (2D Dbl)=dbl[][] []) -> (array=w635:dbl[][])
                n443 = local read "Start Wavelength (nm)"() -> (w631:string)
                n444 = local read "Stop Wavelength (nm)"() -> (w630:string)
                n445 = Index Array(array=w635, index (row)=0) -> (element=w624:dbl[])  [unwired: 1 in]
                n446 = Array Size(array=w624) -> (size(s)=w625:i32)
                n447 = Decimal String To Number(string=w631) -> (number=w626:i32)  [unwired: 2 in, 1 out]
                "Current lambda" <- w626
                n448 = Decimal String To Number(string=w630) -> (number=w629:i32)  [unwired: 2 in, 1 out]
                n449 = Initialize Array(0.0 ("element"), w625) -> (w632:dbl[])
                n450 = Subtract(x=w629, y=w626) -> (x-y=w628:i32)
                n451 = Divide(x=w628, y=w625) -> (x/y=→"data step":dbl)
              }
              frame #1 {
                n452 = for {
                  N: w683 -> [_]
                  shift-right: [w684] -> _
                  shift-left: w682 -> [w685]
                  tunnel: [w684] -> w680
                  i -> [w686]
                  n453 = flat-sequence {
                    tunnel: w685 -> [w690]
                    tunnel: w686 -> [w689]
                    tunnel: [w687] -> w684
                    frame #0 {
                      n454 = local read "Current lambda"() -> (w688:dbl)
                      n455 = Replace Array Subset(array=w690, new element=w688, index=w689) -> (w687:dbl[])
                      "Numeric" <- w689
                    }
                    frame #1 {
                      n456 = local read "Current lambda"() -> (w693:dbl)
                      n457 = local read "data step"() -> (w692:dbl)
                      n458 = Add(x=w693, y=w692) -> (x+y=w691:dbl)
                      n459 = local write "Current lambda"(w691) -> ()
                    }
                  }
                }
              }
              frame #2 {
                n460 = Bundle(w706, "array type (2D Dbl)"=w707) -> (→"Spectrum Readout":cluster{dbl[], "array type (2D Dbl)":dbl[]})  [unwired: 1 in]
                n461 = local read "Current Step Delay"() -> (w699:dbl)
                n462 = local read "FWHM (nm)"() -> (w696:string)
                n463 = local read "Spectrum Measurement Recipe ID"() -> (w701:dbl)
                n464 = local read "Peak Intensity (dBm)"() -> (w702:string)
                n465 = local read "Processing Recipe ID"() -> (w700:dbl)
                n466 = local read "Peak Wavelength (nm)"() -> (w703:string)
                n467 = local read "Temp Setpoint"() -> (w695:string)
                n468 = Number To Decimal String(number=w699) -> (decimal integer string=w698:string)  [unwired: 1 in]
                n469 = local read "Spectrum Parameters"() -> (w704:T3)
                n470 = Decimal String To Number(string=w695) -> (number=w694:i32)  [unwired: 2 in, 1 out]
                n471 = Bundle By Name(cluster=w704, "Peak Wavelengh (dbm)"=w703, "Peak Power (dbm)"=w702, "FWHM (nm)"=w696, "Input Current (mA)"=w698, "Measurement Recipe ID"=w701, "Processing Recipe ID"=w700, "Temperature"=w694) -> (w697:T3)
                n472 = local write "Spectrum Parameters"(w697) -> ()
                "Wavelength Array" <- w706
                "intensity array" <- w707
              }
            }
          }
          frame "stepper fine alignment" {
            n473 = local read "vi path stepper fine"() -> (w709:path)
            n474 = Open VI Reference(vi path=w709) -> (vi reference=w708:refnum<vi>)  [unwired: 5 in, 1 out]
            n475 = invoke on="Sub Panel" class="SubPanel" method="Insert VI"("VI Ref"=w708) -> ()  [unwired: 3 in, 4 out]
            n476 = invoke class="VI" method="Run VI"(reference=w708) -> ()  [unwired: 4 in, 5 out]
            n477 = case shown="True" FALSE {
              frame False {
              }
              frame True {
                n478 = flat-sequence {
                  frame #0 {
                    n479 = local read "Thorlabs PM100 VISA"() -> (w724:refnum<visa-resource-name>)
                    n480 = local read "Serial Numbers Stepper Motors"() -> (w725:T10)
                    n481 = local read "Stepper X Axis"() -> (w714:refnum<k7>)
                    n482 = local write "Status"("aligning steppers..." ("Status")) -> ()
                    n483 = call "NanoMAX300 Align Fiber Steppers.vi"("Serial Numbers Stepper Motors"=w725, "Current Motor"=w714, "Thorlabs PM100 VISA"=w724) -> ("Y profile"=w716:T9, "Z Profile"=w717:T9, "X Profile"=w715:T9, "max power Y (mW)"=w718:dbl, "Y Position at Max Power (mm)"=w719:sgl, "max Power X (mW)"=w723:dbl, "X Position at max power (mm)"=w722:sgl, "Z Position at Max Power (mm)"=w721:sgl, "max power Z (mW)"=w720:dbl)  [unwired: 4 in]
                    n484 = local write "X Axis Profile"(w715) -> ()
                    n485 = local write "Position of Max Power X"(w722) -> ()
                    n486 = local write "Position of Max Power Y"(w719) -> ()
                    n487 = local write "Position of Max Power Z"(w721) -> ()
                    n488 = local write "Z Axis Profile"(w717) -> ()
                    n489 = local write "Max Power Y"(w718) -> ()
                    n490 = local write "Max Power Z"(w720) -> ()
                    n491 = local write "Max Power X"(w723) -> ()
                    n492 = local write "Y Axis Profile"(w716) -> ()
                  }
                  frame #1 {
                    n493 = local write "Status"("idle" ("Status")) -> ()
                  }
                }
              }
            }
          }
          frame "piezo fine alignment" {
            n494 = flat-sequence {
              tunnel: [w731] -> w727
              tunnel: w727 -> [w735]
              frame #0 {
                n495 = local read "vi path piezosfine"() -> (w734:path)
                n496 = Open VI Reference(vi path=w734) -> (vi reference=w733:refnum<vi>)  [unwired: 5 in, 1 out]
                n497 = invoke class="VI" method="Run VI"(reference=w733, "Wait until done"=TRUE ("Wait Until Done")) -> (reference out=w731:refnum<vi>)  [unwired: 3 in, 4 out]
                n498 = invoke on="Sub Panel" class="SubPanel" method="Insert VI"("VI Ref"=w731) -> ()  [unwired: 3 in, 4 out]
              }
              frame #1 {
                n499 = Close Reference(reference=w735) -> ()  [unwired: 1 in, 1 out]
              }
            }
            n500 = case shown="True" FALSE {
              frame False {
              }
              frame True {
                n501 = flat-sequence {
                  frame #0 {
                    n502 = local read "Serial Numbers Piezo"() -> (w747:T10)
                    n503 = local read "Thorlabs PM100 VISA"() -> (w740:refnum<visa-resource-name>)
                    n504 = call "NanoMAX300 Align Fiber Piezos.vi"("Serial Numbers Piezo"=w747, "PM100 Visa"=w740) -> ("x pos"=w746:sgl, "max value x"=w744:dbl, "z pos"=w745:sgl, "Y Profile"=w738:T9, "X Profile"=w739:T9, "Z Profile"=w737:T9, "max value Y"=w741:dbl, "y pos"=w742:sgl, "max value z"=w743:dbl)  [unwired: 7 in, 2 out]
                    n505 = local write "Status"("piezo aligning..." ("Status")) -> ()
                    n506 = local write "X Axis Profile"(w739) -> ()
                    n507 = local write "Z Axis Profile"(w737) -> ()
                    n508 = local write "Y Axis Profile"(w738) -> ()
                    n509 = local write "Position of Max Power Y"(w742) -> ()
                    n510 = local write "Position of Max Power Z"(w745) -> ()
                    n511 = local write "Position of Max Power X"(w746) -> ()
                    n512 = local write "Max Power X"(w744) -> ()
                    n513 = local write "Max Power Y"(w741) -> ()
                    n514 = local write "Max Power Z"(w743) -> ()
                  }
                  frame #1 {
                    n515 = local write "Status"("idle" ("Status")) -> ()
                  }
                }
              }
            }
          }
          frame "find peak" {
            n516 = local read "vi find peak"() -> (w750:path)
            n517 = Open VI Reference(vi path=w750) -> (vi reference=w749:refnum<vi>)  [unwired: 5 in, 1 out]
            n518 = invoke class="VI" method="Run VI"(reference=w749) -> ()  [unwired: 4 in, 5 out]
          }
          frame "update wafer info" {
            n519 = local read "WaferInfo"() -> (w762:T5)
            n520 = local read "DeviceInfo"() -> (w759:T2)
            n521 = Unbundle By Name(w762) -> ("WaferName"=w761:string)
            n522 = Unbundle By Name(w759) -> ("Cavity Length (um)"=w758:string, "Cavity Width (um)"=w757:string, "X Position"=w756:string)
            n523 = call "getDB Wafer Info.vi"("Wafer Name"=w761) -> ("WaferInfo"=w760:T5)  [unwired: 9 in, 1 out]
            n524 = call "getDB Laser Info.vi"("x position"=w756, "width (um)"=w757, "length (um)"=w758) -> ("Part Name"=w754:string)  [unwired: 8 in]
            n525 = local read "DeviceInfo"() -> (w755:T2)
            n526 = Bundle By Name(cluster=w755, "Part Name"=w754) -> (w753:T2)
            n527 = local write "WaferInfo"(w760) -> ()
            n528 = local write "DeviceInfo"(w753) -> ()
          }
          frame "Home Stage" {
            n529 = flat-sequence {
              frame #0 {
                n530 = local read "Serial Numbers Stepper Motors"() -> (w777:T10)
                n531 = local read "Stepper Refs"() -> (w776:refnum<k7>[])
                n532 = Unbundle By Name(w777) -> ("MotorA HWSerialNum"=w773:i32, "Motor B HWSerialNum"=w772:i32, "Motor C HWSerialNum"=w771:i32)
                n533 = local write "Status"("homing..." ("Status")) -> ()
                n534 = Index Array(array=w776, index=0) -> (element=w770:refnum<k7>)
                n535 = Index Array(array=w776, index=1) -> (element=w769:refnum<k7>)
                n536 = Index Array(array=w776, index=2) -> (element=w768:refnum<k7>)
                n537 = call "NanoMAX300 Move Home.vi"("Serial number"=w773, "Automation Refnum in"=w770) -> ()  [unwired: 10 in]
                n538 = call "NanoMAX300 Move Home.vi"("Serial number"=w772, "Automation Refnum in"=w769) -> ()  [unwired: 10 in]
                n539 = call "NanoMAX300 Move Home.vi"("Serial number"=w771, "Automation Refnum in"=w768) -> ()  [unwired: 10 in]
              }
              frame #1 {
                n540 = local write "Status"("home complete" ("Status")) -> ()
              }
            }
          }
          frame "update temptronics" {
            n541 = flat-sequence {
              tunnel: [w785] -> w782
              tunnel: [w784] -> w781
              tunnel: w782 -> [w797]
              tunnel: w781 -> [w798]
              frame #0 {
                n542 = Concatenate Strings("RS" ("string"), "Temp Setpoint") -> (w786:string)
                n543 = VISA Write(VISA resource name="Temptronic VISA", write buffer=w786, error in (no error)=errorcluster {"status"=FALSE, "code"=0, "source"=""}) -> (VISA resource name out=w784:refnum<visa-resource-name>, error out=w785:errorcluster)  [unwired: 1 out]
              }
              frame #1 {
                n544 = VISA Write(VISA resource name=w798, write buffer="ST", error in (no error)=w797) -> (VISA resource name out=w795:refnum<visa-resource-name>, return count=w793:u32, error out=w794:errorcluster)
                n545 = VISA Read(VISA resource name=w795, byte count=w793, error in (no error)=w794) -> (read buffer=→"Current Temp":string, error out=w791:errorcluster)  [unwired: 2 out]
                n546 = local write "Instrument Errors"(w791) -> ()
              }
            }
          }
          frame "add to temp list" {
            n547 = property on="TEMP LIST" class="LstBox (strict)"() -> ("Item Names"=w801:string[])  [unwired: 2 in, 2 out]
            n548 = Build Array (concatenate)(w801, "TEMP DESIRED") -> (w799:string[])
            n549 = property on="TEMP LIST" class="LstBox (strict)"("Item Names"=w799) -> ()  [unwired: 2 in, 2 out]
          }
          frame "clear temp list" {
            n550 = property on="TEMP LIST" class="LstBox (strict)"("Item Names"=string[] []) -> ()  [unwired: 2 in, 2 out]
          }
          frame "remove from temp list" {
            n551 = property on="TEMP LIST" class="LstBox (strict)"() -> ("Item Names"=w808:string[])  [unwired: 2 in, 2 out]
            n552 = local read "TEMP LIST"() -> (w809:i32)
            n553 = Delete From Array(array=w808, index=w809) -> (array with subset deleted=w807:string[])  [unwired: 1 in, 1 out]
            n554 = property on="TEMP LIST" class="LstBox (strict)"("Item Names"=w807) -> ()  [unwired: 2 in, 2 out]
          }
          frame "begin temp series" {
            n555 = flat-sequence {
              frame #0 {
                w814 = cluster{dbl[], dbl[]}[] [] ("Current v. Power")
                n556 = property on="TEMP LIST" class="LstBox (strict)"() -> ("Item Names"=w821:string[])  [unwired: 2 in, 2 out]
                n557 = Get Date/Time In Seconds() -> ()  [unwired: 1 out]
                n558 = local read "Arroyo VISA"() -> (w820:refnum<visa-resource-name>)
                n559 = local write "P array"(dbl[] [] ("V Array")) -> ()
                n560 = local write "I Array"(dbl[] [] ("I Array")) -> ()
                n561 = property on="Current v. Power" class="XYGraph (strict)"("Value"=w814) -> ()  [unwired: 2 in, 2 out]
                n562 = property on="Voltage v. Current" class="XYGraph (strict)"("Value"=w814) -> ()  [unwired: 2 in, 2 out]
                n563 = call <instrlib>:"Arroyo LAS OUTPUT.vi"("Laser Output Enable"=TRUE, "VISA resource name"=w820) -> ()  [unwired: 1 in, 2 out]
                n564 = for {
                  tunnel: w821 -> [_] mode=indexing
                  tunnel: [w826] -> w816 mode=indexing
                  tunnel: [w825] -> w815 mode=indexing
                  i -> [w824]
                  n565 = flat-sequence {
                    tunnel: w824 -> [w830]
                    tunnel: [w867] -> w829
                    tunnel: [w868] -> w828
                    tunnel: [w869] -> w827
                    tunnel: [w876] -> w826
                    tunnel: [w875] -> w825
                    tunnel: w824 -> [w871]
                    tunnel: w829 -> [w912]
                    tunnel: w828 -> [w911]
                    tunnel: w827 -> [w910]
                    tunnel: [w980] -> w823
                    tunnel: [w979] -> w822
                    tunnel: w823 -> [w997]
                    tunnel: w822 -> [w996]
                    frame #0 {
                      n566 = property on="TEMP LIST" class="LstBox (strict)"() -> ("Item Names"=w832:string[])  [unwired: 2 in, 2 out]
                      n567 = Index Array(array=w832, index=w830) -> (element=w831:string)
                      n568 = local write "Temp Setpoint"(w831) -> ()
                    }
                    frame #1 {
                      n569 = local read "Arroyo VISA"() -> (w834:refnum<visa-resource-name>)
                      n570 = while {
                        stop <- w837 stop-if-true
                        # "This Loop Updates the Temperature, and stops when temperature reached setpoint"
                        n571 = call "Time Delay4"() -> ()  [unwired: 11 in, 1 out]
                        n572 = local read "Temp Setpoint"() -> (w835:string)
                        n573 = local read "Temptronic VISA"() -> (w842:refnum<visa-resource-name>)
                        n574 = Concatenate Strings("RS" ("string"), w835) -> (w848:string)
                        n575 = local write "Status"("Adjusting Temperature..." ("Status")) -> ()
                        n576 = VISA Write(VISA resource name=w842, write buffer=w848, error in (no error)=errorcluster {"status"=FALSE, "code"=0, "source"=""}) -> (VISA resource name out=w841:refnum<visa-resource-name>, error out=w840:errorcluster)  [unwired: 1 out]
                        n577 = VISA Write(VISA resource name=w841, write buffer="ST", error in (no error)=w840) -> (VISA resource name out=w846:refnum<visa-resource-name>, return count=w844:u32, error out=w845:errorcluster)
                        n578 = VISA Read(VISA resource name=w846, byte count=w844, error in (no error)=w845) -> (read buffer=w838:string, error out=w839:errorcluster)  [unwired: 2 out]
                        n579 = Equal?(x=w838, y=w835) -> (x = y?=w837:bool)
                        n580 = local write "Current Temp"(w838) -> ()
                        n581 = local write "Instrument Errors"(w839) -> ()
                      }
                      n582 = call <instrlib>:"Arroyo LAS LDI.vi"("Laser Current Setpoint"=0.0, "VISA resource name"=w834) -> ()  [unwired: 1 in, 2 out]
                    }
                    frame #2 {
                      n583 = call "Time Delay6"("Delay Time (s)"=1.0) -> ()  [unwired: 10 in, 1 out]
                      n584 = local read "Start Current"() -> (w864:dbl)
                      n585 = local read "Start Current"() -> (w858:dbl)
                      n586 = local read "End Current"() -> (w865:dbl)
                      n587 = local read "Counts per Data Point"() -> (w857:i32)
                      n588 = local read "Arroyo VISA"() -> (w859:refnum<visa-resource-name>)
                      n589 = local read "Time per Count (s)"() -> (w856:dbl)
                      n590 = local read "Step Size"() -> (w862:dbl)
                      n591 = local read "Current Step Delay"() -> (w850:dbl)
                      n592 = local write "Current Setpoint"(w858) -> ()
                      n593 = call <instrlib>:"Arroyo LAS LDI.vi"("Laser Current Setpoint"=w858, "VISA resource name"=w859) -> ()  [unwired: 1 in, 2 out]
                      n594 = Subtract(x=w865, y=w864) -> (x-y=w863:dbl)
                      n595 = Divide(x=w863, y=w862) -> (x/y=w861:dbl)
                      n596 = Multiply(x=w857, y=w856) -> (x*y=w855:dbl)
                      n597 = Add(x=w855, y=w850) -> (x+y=w854:dbl)
                      n598 = Add(x=w861, y=1.0) -> (x+y=w853:dbl)
                      n599 = Multiply(x=w853, y=w854) -> (x*y=→"Estimated Sweep Time":dbl)
                      n600 = local write "# Data Points"(w853) -> ()
                    }
                    frame #3 {
                      n601 = local read "Continuous Wave"() -> (w866:bool)
                      n602 = local read "Current Temp"() -> (w874:string)
                      n603 = local write "Status"("sweeping..." ("Status")) -> ()
                      n604 = case shown="True" w866 {
                        tunnel: [w880 w903] -> w869
                        tunnel: [w881 w902] -> w868
                        tunnel: [w882 w901] -> w867
                        frame False {
                          n605 = control-ref of="Measured Average Current"() -> (w878:refnum<vi>)
                          n606 = control-ref of="Calculated Peak Current"() -> (w879:refnum<vi>)
                          n607 = local read "Delay Width (ms)"() -> (w895:dbl)
                          n608 = local read "Pulse Width (ms)"() -> (w893:dbl)
                          n609 = local read "Quantum Composers VISA"() -> (w898:refnum<visa-resource-name>)
                          n610 = local read "Counts per Data Point"() -> (w884:i32)
                          n611 = local read "Thorlabs PM100 VISA"() -> (w897:refnum<visa-resource-name>)
                          n612 = local read "Current Step Delay"() -> (w883:dbl)
                          n613 = local read "Time per Count (s)"() -> (w886:dbl)
                          n614 = local read "# Data Points"() -> (w896:dbl)
                          n615 = local read "Start Current"() -> (w888:dbl)
                          n616 = local read "End Current"() -> (w887:dbl)
                          n617 = local read "Duty Cycle"() -> (w889:dbl)
                          n618 = local read "Step Size"() -> (w885:dbl)
                          n619 = Divide(x=w895, y=1000.0) -> (x/y=w890:dbl)
                          n620 = Divide(x=w893, y=1000.0) -> (x/y=w894:dbl)
                          n621 = call "QC Current_Voltage Sweep.vi"("Quantum Composers VISA"=w898, "Thorlabs PM100 VISA"=w897, "Delay (10 msec)"=w890, "# Data Points"=w896, "Width (10 msec)"=w894, "Duty Cycle"=w889, "Step Size"=w885, "Start Current"=w888, "Counts per Data Point"=w884, "End Current"=w887, "Current Step Time"=w883, "Time per Count (s)"=w886, "Measured Current Ref"=w878, "Peak Current Ref"=w879) -> ("V Array"=w882:dbl[], "I Array"=w881:dbl[], "P Array"=w880:dbl[])  [unwired: 3 in]
                        }
                        frame True {
                          n622 = control-ref of="Measured Average Current"() -> (w900:refnum<vi>)
                          n623 = control-ref of="Calculated Peak Current"() -> (w899:refnum<vi>)
                          n624 = local read "Counts per Data Point"() -> (w905:i32)
                          n625 = local read "# Data Points"() -> (w909:dbl)
                          n626 = local read "Start Current"() -> (w908:dbl)
                          n627 = local read "Arroyo VISA"() -> (w904:refnum<visa-resource-name>)
                          n628 = local read "End Current"() -> (w907:dbl)
                          n629 = local read "Step Size"() -> (w906:dbl)
                          n630 = call "Arroyo Current Sweep.vi"("Arroyo VISA"=w904, "Counts per Data Point"=w905, "Step Size"=w906, "End Current"=w907, "Start Current"=w908, "# Data Points"=w909, "Measured Current Measured Refnum"=w900, "Peak Current Measured Refnum"=w899) -> ("Voltage"=w901:dbl[], "Current"=w902:dbl[], "Power Array"=w903:dbl[])  [unwired: 9 in]
                        }
                      }
                      n631 = Concatenate Strings(w874, " C" ("string")) -> (w872:string)
                      n632 = property on="Current v. Power" class="XYGraph (strict)"("Active Plot"=w871, "Plot.Plot Name"=w872) -> ()  [unwired: 2 in, 2 out]
                      n633 = property on="Voltage v. Current" class="XYGraph (strict)"("Active Plot"=w871, "Plot.Plot Name"=w872) -> ()  [unwired: 2 in, 2 out]
                      n634 = local write "I Array"(w868) -> ()
                      n635 = local write "V Array"(w867) -> ()
                      n636 = Build Array(w867, w868, w869) -> (→"LIV Array":dbl[][])
                      n637 = Bundle("Current"=w868, "Power Array"=w869) -> (w875:cluster{"Current":dbl[], "Power Array":dbl[]})  [unwired: 1 out]
                      n638 = local write "P array"(w869) -> ()
                      n639 = Bundle("Voltage"=w867, "Current"=w868) -> (w876:cluster{"Voltage":dbl[], "Current":dbl[]})  [unwired: 1 out]
                    }
                    frame #4 {
                      n640 = call "Caucluate Parameters LIV.vi"("Voltage Array"=w912, "I Array"=w911, "P Array"=w910) -> ("Current @ Max Power"=w920:dbl, "Max Power (mW)"=w919:dbl, "slope efficincy"=w918:dbl, "DQE"=w917:dbl, "energy/photon (eV)"=w916:dbl, "Least Squares Residue"=w915:dbl, "Threshold Voltage (V)"=w913:dbl, "Threshold Current (mA)"=w914:dbl)  [unwired: 5 in]
                      n641 = local write "DQE"(w917) -> ()
                      n642 = local write "Current @ Max Power"(w920) -> ()
                      n643 = local write "Max Power (mW)"(w919) -> ()
                      n644 = local write "slope efficincy"(w918) -> ()
                      n645 = local write "energy/photon (eV)"(w916) -> ()
                      n646 = local write "Least Squares Residue"(w915) -> ()
                      n647 = local write "Threshold Current (mA)"(w914) -> ()
                      n648 = local write "Threshold Voltage (V)"(w913) -> ()
                    }
                    frame #5 {
                      n649 = local read "Pulse Width (ms)"() -> (w928:dbl)
                      n650 = local read "Temp Setpoint"() -> (w925:string)
                      n651 = local read "Threshold Current (mA)"() -> (w924:dbl)
                      n652 = local read "Threshold Voltage (V)"() -> (w923:dbl)
                      n653 = local read "LIV Parameters"() -> (w926:T4)
                      n654 = local read "DQE"() -> (w922:dbl)
                      n655 = Decimal String To Number(string=w925) -> (number=w921:i32)  [unwired: 2 in, 1 out]
                      n656 = Multiply(x=1000.0, y=w928) -> (x*y=w936:dbl)
                      n657 = Bundle By Name(cluster=w926, "Threshold Current (mA)"=w924, "Threshold Voltage (V)"=w923, "Slope Efficiency"=w922, "Temperature"=w921) -> (w927:T4)
                      n658 = local read "Counts per Data Point"() -> (w933:i32)
                      n659 = local read "Time per Count (s)"() -> (w934:dbl)
                      n660 = local read "Start Current"() -> (w930:dbl)
                      n661 = local read "End Current"() -> (w931:dbl)
                      n662 = local read "Duty Cycle"() -> (w935:dbl)
                      n663 = local read "Step Size"() -> (w932:dbl)
                      n664 = Number To Exponential String(number=w936) -> (E-format string=w943:string)  [unwired: 3 in]
                      n665 = Number To Exponential String(number=w930) -> (E-format string=w937:string)  [unwired: 3 in]
                      n666 = Number To Exponential String(number=w931) -> (E-format string=w938:string)  [unwired: 3 in]
                      n667 = Number To Exponential String(number=w932) -> (E-format string=w939:string)  [unwired: 3 in]
                      n668 = Number To Exponential String(number=w933) -> (E-format string=w940:string)  [unwired: 3 in]
                      n669 = Number To Exponential String(number=w934) -> (E-format string=w941:string)  [unwired: 3 in]
                      n670 = Number To Exponential String(number=w935) -> (E-format string=w942:string)  [unwired: 3 in]
                      n671 = local write "LIV Parameters"(w927) -> ()
                      n672 = call "Check for LIV Measurement Recipe.vi"("pulse width us"=w943, "time per measurement s"=w941, "end current"=w938, "duty cycle"=w942, "points averaged per measurement"=w940, "step size"=w939, "start current"=w937) -> ("Measurement ID"=w946:string)  [unwired: 3 in]
                      n673 = Equal?(x=w946, y="") -> (x = y?=w945:bool)
                      n674 = case shown="True" w945 {
                        tunnel: w946 -> [w948 _]
                        frame False {
                          n675 = Decimal String To Number(string=w948) -> (number=w947:i32)  [unwired: 2 in, 1 out]
                          n676 = local read "LIV Parameters"() -> (w950:T4)
                          n677 = Bundle By Name(cluster=w950, "Measurement Recipe ID"=w947) -> (w949:T4)
                          n678 = local write "LIV Parameters"(w949) -> ()
                        }
                        frame True {
                          n679 = local read "Pulse Width (ms)"() -> (w964:dbl)
                          n680 = Multiply(x=1000.0, y=w964) -> (x*y=w972:dbl)
                          n681 = local read "Counts per Data Point"() -> (w969:i32)
                          n682 = local read "Time per Count (s)"() -> (w970:dbl)
                          n683 = local read "# Data Points"() -> (w958:dbl)
                          n684 = local read "Start Current"() -> (w966:dbl)
                          n685 = local read "End Current"() -> (w967:dbl)
                          n686 = local read "Duty Cycle"() -> (w971:dbl)
                          n687 = local read "Step Size"() -> (w968:dbl)
                          n688 = Number To Exponential String(number=w971) -> (E-format string=w955:string)  [unwired: 3 in]
                          n689 = Number To Exponential String(number=w969) -> (E-format string=w956:string)  [unwired: 3 in]
                          n690 = Number To Exponential String(number=w966) -> (E-format string=w962:string)  [unwired: 3 in]
                          n691 = Number To Exponential String(number=w967) -> (E-format string=w961:string)  [unwired: 3 in]
                          n692 = Number To Exponential String(number=w968) -> (E-format string=w960:string)  [unwired: 3 in]
                          n693 = Number To Exponential String(number=w958) -> (E-format string=w959:string)  [unwired: 3 in]
                          n694 = Number To Exponential String(number=w970) -> (E-format string=w957:string)  [unwired: 3 in]
                          n695 = Number To Exponential String(number=w972) -> (E-format string=w963:string)  [unwired: 3 in]
                          n696 = local read "LIV Parameters"() -> (w954:T4)
                          n697 = call "Insert New LIV Recipe into db.vi"("pulse width us"=w963, "duty cycle"=w955, "time per measurement s"=w957, "points averaged per measurement"=w956, "# data points"=w959, "step size"=w960, "end current"=w961, "start current"=w962) -> ("New Measurement ID"=w952:string)  [unwired: 3 in]
                          n698 = Decimal String To Number(string=w952) -> (number=w951:i32)  [unwired: 2 in, 1 out]
                          n699 = Bundle By Name(cluster=w954, "Measurement Recipe ID"=w951) -> (w953:T4)
                          n700 = local write "LIV Parameters"(w953) -> ()
                        }
                      }
                    }
                    frame #6 {
                      n701 = local read "Threshold Current (mA)"() -> (w987:dbl)
                      n702 = local read "Temp Setpoint"() -> (w988:string)
                      n703 = local read "Threshold Voltage (V)"() -> (w986:dbl)
                      n704 = local read "LIV Parameters"() -> (w989:T4)
                      n705 = Decimal String To Number(string=w988) -> (number=w984:i32)  [unwired: 2 in, 1 out]
                      n706 = local read "DeviceInfo"() -> (w977:T2)
                      n707 = local read "WaferInfo"() -> (w983:T5)
                      n708 = local read "DQE"() -> (w985:dbl)
                      n709 = Bundle By Name(cluster=w989, "Threshold Current (mA)"=w987, "Threshold Voltage (V)"=w986, "Slope Efficiency"=w985, "Temperature"=w984) -> (w979:T4)
                      "LIV Parameters" <- w979
                      n710 = Unbundle By Name(w983) -> ("WaferName"=w982:string)
                      n711 = Unbundle By Name(w977) -> ("Part Name"=w976:string)
                      n712 = local read "Sweep save path"() -> (w978:path)
                      n713 = local read "Dates"() -> (w975:T1)
                      n714 = Get Date/Time In Seconds() -> (seconds since 1Jan1904=w974:timestamp)
                      n715 = Bundle By Name(cluster=w975, "Measurement Date"=w974) -> (w973:T1)
                      n716 = local write "Dates"(w973) -> ()
                      n717 = call "get Flash FileName .vi"("Time"=w974, "Device Name"=w976, "Operator"="Operator", "Wafer Name"=w982, "FineTest save path"=w978) -> ("appended path"=w980:path)  [unwired: 6 in]
                    }
                    frame #7 {
                      n718 = local read "LIV Measurement Comments"() -> (w991:string)
                      n719 = local read "DeviceInfo"() -> (w992:T2)
                      n720 = local read "WaferInfo"() -> (w994:T5)
                      n721 = local read "Operator"() -> (w993:string)
                      n722 = local read "LIV Array"() -> (w995:dbl[][])
                      n723 = local read "Dates"() -> (w990:T1)
                      n724 = call "WriteFlashFile EELS.vi"("Input File Path"=w997, "LIV Parameters"=w996, "LIV Measurement Comments"=w991, "Operator"=w993, "WaferInfo"=w994, "Dates"=w990, "DeviceInfo"=w992, "LIV array"=w995) -> ()  [unwired: 7 in, 1 out]
                    }
                  }
                }
                "Voltage v. Current" <- w816
                "Current v. Power" <- w815
              }
              frame #1 {
                w1011 = "25" ("string")
                n725 = local read "Temptronic VISA"() -> (w1008:refnum<visa-resource-name>)
                n726 = local write "Temp Setpoint"(w1011) -> ()
                n727 = Concatenate Strings("RS" ("string"), w1011) -> (w1006:string)
                n728 = VISA Write(VISA resource name=w1008, write buffer=w1006, error in (no error)=errorcluster {"status"=FALSE, "code"=0, "source"=""}) -> (VISA resource name out=w1009:refnum<visa-resource-name>, error out=w1010:errorcluster)  [unwired: 1 out]
                n729 = local read "Arroyo VISA"() -> (w1000:refnum<visa-resource-name>)
                n730 = call <instrlib>:"Arroyo LAS OUTPUT.vi"("Laser Output Enable"=FALSE, "VISA resource name"=w1000) -> ()  [unwired: 1 in, 2 out]
                n731 = VISA Write(VISA resource name=w1009, write buffer="ST", error in (no error)=w1010) -> (VISA resource name out=w1003:refnum<visa-resource-name>, return count=w1002:u32, error out=w1001:errorcluster)
                n732 = local write "Status"("idle" ("Status")) -> ()
                n733 = VISA Read(VISA resource name=w1003, byte count=w1002, error in (no error)=w1001) -> (read buffer=w1012:string)  [unwired: 3 out]
                n734 = local write "Current Temp"(w1012) -> ()
              }
            }
          }
          frame "cw change" {
            n735 = local read "Continuous Wave"() -> (w1014:bool)
            n736 = Not(x=w1014) -> (.not. x?=w1013:bool)
            n737 = case shown="True" w1013 {
              frame False {
                w1017 = 0 items=["System (To)", "Channel A", "Channel B", "Channel C", "Channel D", "Channel E", "Channel F", "Channel G", "Channel H"] ("Channel (1:Chan A)")
                w1020 = 1.0 ("Duty Cycle (Update in Settings)")
                n738 = local read "Quantum Composers VISA"() -> (w1019:refnum<visa-resource-name>)
                n739 = call <instrlib>:"Enable Chan-Sys.vi"("Channel (1:Chan A)"=w1017, "State (T:Enabled)"=FALSE, "VISA resource name"=w1019) -> ()  [unwired: 7 in, 2 out]
                n740 = local write "Duty Cycle (Update in Settings)"(w1020) -> ()
                n741 = local write "Duty Cycle"(w1020) -> ()
              }
              frame True {
                w1021 = 0 items=["System (To)", "Channel A", "Channel B", "Channel C", "Channel D", "Channel E", "Channel F", "Channel G", "Channel H"] ("Channel (1:Chan A)")
                n742 = local read "Quantum Composers VISA"() -> (w1023:refnum<visa-resource-name>)
                n743 = local read "Pulse Width (ms)"() -> (w1025:dbl)
                n744 = local read "Delay Width (ms)"() -> (w1026:dbl)
                n745 = Add(x=w1025, y=w1026) -> (x+y=w1027:dbl)
                n746 = Divide(x=w1025, y=w1027) -> (x/y=w1024:dbl)
                n747 = call <instrlib>:"Enable Chan-Sys.vi"("Channel (1:Chan A)"=w1021, "State (T:Enabled)"=TRUE, "VISA resource name"=w1023) -> ()  [unwired: 7 in, 2 out]
                n748 = local write "Duty Cycle (Update in Settings)"(w1024) -> ()
                n749 = local write "Duty Cycle"(w1024) -> ()
              }
            }
          }
          frame "select processing recipe" {
            n750 = call "getDB EELS Processing Recipes.vi"() -> ("Desired ID"=w1030:string, "Current Recipe"=w1028:T7)  [unwired: 10 in]
            n751 = local write "Current Processing Recipe"(w1028) -> ()
            n752 = Decimal String To Number(string=w1030) -> (number=w1029:i32)  [unwired: 2 in, 1 out]
            n753 = local read "LIV Parameters"() -> (w1032:T4)
            n754 = Bundle By Name(cluster=w1032, "Processing Recipe ID"=w1029) -> (w1031:T4)
            n755 = local write "LIV Parameters"(w1031) -> ()
          }
        }
      }
      n756 = while {
        shift-right: [w1038] -> w39
        shift-left: w35 -> [w1037]
        shift-right: [w1036] -> w37
        shift-left: w36 -> [w1039]
        stop <- w1035 stop-if-true
        n757 = event shown="[25] \"stop\": Value Change" {
          selector: _ -> [_ _ _ _ _ _ _ _ _ _ _ _ _ _ _ _ _ _ _ _ _ _ _ _ _ _]
          dyn-events: _ -> [_ _ _ _ _ _ _ _ _ _ _ _ _ _ _ _ _ _ _ _ _ _ _ _ _ _]
          timeout: _ -> [_ _ _ _ _ _ _ _ _ _ _ _ _ _ _ _ _ _ _ _ _ _ _ _ _ _]
          tunnel: w1039 -> [w1044 w1047 w1053 w1057 w1062 w1068 w1070 w1077 w1081 w1087 w1092 w1098 w1103 w1107 w1110 w1117 w1123 w1128 w1131 w1138 w1141 w1147 w1151 w1156 w1161 w1167]
          tunnel: w1037 -> [w1043 w1048 w1054 w1059 w1063 w1067 w1071 w1079 w1084 w1089 w1094 w1099 w1102 w1108 w1111 w1119 w1124 w1129 w1133 w1139 w1144 w1149 w1154 w1159 w1164 w1168]
          tunnel: [w1041 w1046 w1052 w1056 w1060 w1065 w1072 w1076 w1082 w1086 w1091 w1096 w1100 w1105 w1112 w1116 w1121 w1126 w1130 w1136 w1142 w1146 w1152 w1157 w1162 w1165] -> w1036
          tunnel: [w1040 w1045 w1051 w1058 w1061 w1066 w1073 w1078 w1083 w1088 w1093 w1097 w1101 w1106 w1113 w1118 w1122 w1127 w1132 w1137 w1143 w1148 w1153 w1158 w1163 w1166] -> w1038
          tunnel: [_ _ _ _ _ _ _ _ _ _ _ _ _ _ _ _ _ _ _ _ _ _ _ _ _ TRUE] -> w1035
          event Timeout {
            n758 = event-data() -> ()  [unwired: 1 in, 2 out]
            n759 = Enqueue Element(queue=w1043, element="idle", error in (no error)=w1044) -> (queue out=w1040:refnum<queue>, error out=w1041:errorcluster)  [unwired: 1 in, 1 out]
          }
          event Value Change {
            n760 = event-data() -> ()  [unwired: 1 in, 6 out]
            n761 = Enqueue Element(queue=w1048, element="update laser driver", error in (no error)=w1047) -> (queue out=w1045:refnum<queue>, error out=w1046:errorcluster)  [unwired: 1 in, 1 out]
          }
          event "Find Peak": Value Change {
            n762 = event-data() -> ()  [unwired: 1 in, 6 out]
            n763 = Enqueue Element(queue=w1054, element="find peak", error in (no error)=w1053) -> (queue out=w1051:refnum<queue>, error out=w1052:errorcluster)  [unwired: 1 in, 1 out]
          }
          event "update wafer info": Value Change {
            n764 = event-data() -> ()  [unwired: 1 in, 6 out]
            n765 = Enqueue Element(queue=w1059, element="update wafer info", error in (no error)=w1057) -> (queue out=w1058:refnum<queue>, error out=w1056:errorcluster)  [unwired: 1 in, 1 out]
          }
          event "power meter": Value Change {
            n766 = event-data() -> ()  [unwired: 1 in, 6 out]
            n767 = Enqueue Element(queue=w1063, element="update power meter", error in (no error)=w1062) -> (queue out=w1061:refnum<queue>, error out=w1060:errorcluster)  [unwired: 1 in, 1 out]
          }
          event "pulse generator update": Value Change {
            n768 = event-data() -> ()  [unwired: 1 in, 6 out]
            n769 = Enqueue Element(queue=w1067, element="update pulse generator", error in (no error)=w1068) -> (queue out=w1066:refnum<queue>, error out=w1065:errorcluster)  [unwired: 1 in, 1 out]
          }
          event "start sweep": Value Change {
            n770 = event-data() -> ()  [unwired: 1 in, 6 out]
            n771 = Enqueue Element(queue=w1071, element="current sweep", error in (no error)=w1070) -> (queue out=w1073:refnum<queue>, error out=w1072:errorcluster)  [unwired: 1 in, 1 out]
          }
          event "spectrum measuement presets 2": Value Change {
            n772 = event-data() -> ()  [unwired: 1 in, 6 out]
            n773 = Enqueue Element(queue=w1079, element="select spectrum recipe", error in (no error)=w1077) -> (queue out=w1078:refnum<queue>, error out=w1076:errorcluster)  [unwired: 1 in, 1 out]
          }
          event "Enable Manual Stage Control": Value Change {
            n774 = event-data() -> ()  [unwired: 1 in, 6 out]
            n775 = Enqueue Element(queue=w1084, element="enable manual stage control", error in (no error)=w1081) -> (queue out=w1083:refnum<queue>, error out=w1082:errorcluster)  [unwired: 1 in, 1 out]
          }
          event "Move to Loading Position": Value Change {
            n776 = event-data() -> ()  [unwired: 1 in, 6 out]
            n777 = Enqueue Element(queue=w1089, element="move to loading position", error in (no error)=w1087) -> (queue out=w1088:refnum<queue>, error out=w1086:errorcluster)  [unwired: 1 in, 1 out]
          }
          event "Temptronics update": Value Change {
            n778 = event-data() -> ()  [unwired: 1 in, 6 out]
            n779 = Enqueue Element(queue=w1094, element="update temptronics", error in (no error)=w1092) -> (queue out=w1093:refnum<queue>, error out=w1091:errorcluster)  [unwired: 1 in, 1 out]
          }
          event "Home Stepper Motors": Value Change {
            n780 = event-data() -> ()  [unwired: 1 in, 6 out]
            n781 = Enqueue Element(queue=w1099, element="Home Stage", error in (no error)=w1098) -> (queue out=w1097:refnum<queue>, error out=w1096:errorcluster)  [unwired: 1 in, 1 out]
          }
          event "auto align": Value Change {
            n782 = event-data() -> ()  [unwired: 1 in, 6 out]
            n783 = Enqueue Element(queue=w1102, element="Auto Align", error in (no error)=w1103) -> (queue out=w1101:refnum<queue>, error out=w1100:errorcluster)  [unwired: 1 in, 1 out]
          }
          event "Update OSA Settings": Value Change {
            n784 = event-data() -> ()  [unwired: 1 in, 6 out]
            n785 = Enqueue Element(queue=w1108, element="osa settings update", error in (no error)=w1107) -> (queue out=w1106:refnum<queue>, error out=w1105:errorcluster)  [unwired: 1 in, 1 out]
          }
          event "Preform Sweep": Value Change {
            n786 = event-data() -> ()  [unwired: 1 in, 6 out]
            n787 = Enqueue Element(queue=w1111, element="osa sweep", error in (no error)=w1110) -> (queue out=w1113:refnum<queue>, error out=w1112:errorcluster)  [unwired: 1 in, 1 out]
          }
          event "select processing recipe": Value Change {
            n788 = event-data() -> ()  [unwired: 1 in, 6 out]
            n789 = Enqueue Element(queue=w1119, element="select processing recipe", error in (no error)=w1117) -> (queue out=w1118:refnum<queue>, error out=w1116:errorcluster)  [unwired: 1 in, 1 out]
          }
          event "Continuous Wave": Value Change {
            n790 = event-data() -> ()  [unwired: 1 in, 6 out]
            n791 = Enqueue Element(queue=w1124, element="cw change", error in (no error)=w1123) -> (queue out=w1122:refnum<queue>, error out=w1121:errorcluster)  [unwired: 1 in, 1 out]
          }
          event "auto align step fine": Value Change {
            n792 = event-data() -> ()  [unwired: 1 in, 6 out]
            n793 = Enqueue Element(queue=w1129, element="stepper fine alignment", error in (no error)=w1128) -> (queue out=w1127:refnum<queue>, error out=w1126:errorcluster)  [unwired: 1 in, 1 out]
          }
          event "Save Spectrum to File": Value Change {
            n794 = event-data() -> ()  [unwired: 1 in, 6 out]
            n795 = Enqueue Element(queue=w1133, element="save OSA spectrum", error in (no error)=w1131) -> (queue out=w1132:refnum<queue>, error out=w1130:errorcluster)  [unwired: 1 in, 1 out]
          }
          event "measuement presets": Value Change {
            n796 = event-data() -> ()  [unwired: 1 in, 6 out]
            n797 = Enqueue Element(queue=w1139, element="select LIV measurement preset", error in (no error)=w1138) -> (queue out=w1137:refnum<queue>, error out=w1136:errorcluster)  [unwired: 1 in, 1 out]
          }
          event "add temp to list": Value Change {
            n798 = event-data() -> ()  [unwired: 1 in, 6 out]
            n799 = Enqueue Element(queue=w1144, element="add to temp list", error in (no error)=w1141) -> (queue out=w1143:refnum<queue>, error out=w1142:errorcluster)  [unwired: 1 in, 1 out]
          }
          event "auto align piezo fine": Value Change {
            n800 = event-data() -> ()  [unwired: 1 in, 6 out]
            n801 = Enqueue Element(queue=w1149, element="piezo fine alignment", error in (no error)=w1147) -> (queue out=w1148:refnum<queue>, error out=w1146:errorcluster)  [unwired: 1 in, 1 out]
          }
          event "clear list": Value Change {
            n802 = event-data() -> ()  [unwired: 1 in, 6 out]
            n803 = Enqueue Element(queue=w1154, element="clear temp list", error in (no error)=w1151) -> (queue out=w1153:refnum<queue>, error out=w1152:errorcluster)  [unwired: 1 in, 1 out]
          }
          event "remove temp list": Value Change {
            n804 = event-data() -> ()  [unwired: 1 in, 6 out]
            n805 = Enqueue Element(queue=w1159, element="remove from temp list", error in (no error)=w1156) -> (queue out=w1158:refnum<queue>, error out=w1157:errorcluster)  [unwired: 1 in, 1 out]
          }
          event "begin temp series": Value Change {
            n806 = event-data() -> ()  [unwired: 1 in, 6 out]
            n807 = Enqueue Element(queue=w1164, element="begin temp series", error in (no error)=w1161) -> (queue out=w1163:refnum<queue>, error out=w1162:errorcluster)  [unwired: 1 in, 1 out]
          }
          event "stop": Value Change {
            n808 = event-data() -> ()  [unwired: 1 in, 6 out]
            n809 = Enqueue Element(queue=w1168, element="stop", error in (no error)=w1167) -> (queue out=w1166:refnum<queue>, error out=w1165:errorcluster)  [unwired: 1 in, 1 out]
          }
        }
      }
      n810 = Release Queue(queue=w39, force destroy? (F)=TRUE, error in (no error)=w37) -> (error out=→"error out":errorcluster)  [unwired: 2 out]
    }
  }
